vi "nanocal -- nuclear schottky fit V2.vi"() -> ()   [LabVIEW 2020]
uses:
  filename-pattern.ctl
  show-win- control.ctl
  cursor winow.ctl
  3-lorentzian-heat-response action.ctl
  nanocal-goodness-weighting-strategy.ctl
  <vilib>/gmath/NumericalOptimization/stopping criteria.ctl
  cursor window action.ctl
  cursor action.ctl
  2Dwindow.ctl
  publisher action.ctl
  <vilib>/gmath/NumericalOptimization/objective function data.ctl
  filename-action.ctl
  <vilib>/Utility/miscctls.llb/LVMapReplaceAction.ctl
  file -- read-write control.ctl
  array -- freq-voltage transformations action.ctl
  KM_file -- read-write control.ctl
  replace cursor action stack.vi
  Q -- range multiplier -- real -- V2.vi
  Q - not nan and gtr than zero - Real.vi
  Q - not nan -- real.vi
  Q -- check range -- i -- real.vi
  array - smart min max.vi
  3-lorentzian-heat-response -- V3.vi/142dd4c5-f9ed-c64b-bc14-a88e3e2c450a.vi
  3-lorentzian-heat-response -- analytic derivatives V3.vi
  array -- integrate scalar product.vi
  array -- freq-voltage transformations.vi/05c44075-957c-bc42-b6fa-2799d0bc0485.vi
  tale of three indices.vi
  filter -- window span logic.vi
  linear interp iiii- complex - z-omega - divide.vi
  linear interpolation iiii- complex.vi
  containing bix.vi
  3-lorentzian-heat-response.vi/142dd4c5-f9ed-c64b-bc14-a88e3e2c450a.vi
  <vilib>/Array/Sort 2D Array - Pop Stack.vi
  <vilib>/Array/Sort 2D Array - Push Stack.vi
  array -- freq-voltage transformations.vi/05c44075-957c-bc42-b6fa-2799d0bc0485.vi/5dd0d2be-718e-c148-b8fa-e083cdba2843.vi
  array -- freq-voltage transformations.vi/05c44075-957c-bc42-b6fa-2799d0bc0485.vi/095795a0-771d-c341-9fed-d90d2e44c51c.vi
  command stack.vi
  tale of three indices -- check state.vi
  Q -- check range -- i -- integer.vi
  linear interp iiii- complex - z-omega.vi
  line -- complex.vi
  Q - not nan -- integer.vi
  <vilib>/Analysis/baseanly.llb/A x B.vi
  <vilib>/Analysis/baseanly.llb/Complex A x B.vi
  array -- 3-finitediff.vi
  <vilib>/Analysis/polynomials.llb/Multiply Polynomials.vi
  <vilib>/Analysis/polynomials.llb/Multiply Polynomials (DBL).vi
  <vilib>/Analysis/polynomials.llb/Polynomial Roots.vi
  <vilib>/Analysis/polynomials.llb/Polynomial Roots (DBL).vi
  <vilib>/gmath/NumericalOptimization/Quasi Newton.vi
  <vilib>/Analysis/Matrix/Numeric/Conversions/Array To Matrix.vi
  <vilib>/Analysis/Matrix/Numeric/Conversions/Array To Matrix - RA2.vi
  <vilib>/Analysis/baseanly.llb/Inverse Matrix.vi
  <vilib>/Analysis/baseanly.llb/Real Inverse Matrix.vi
  <vilib>/Comparison/Less/Less Functor/Less Functor.lvclass
  <vilib>/gmath/NI_Gmath.lvlib
panel:
  in  "strings stuff tab":T1(tab)
  in  "string IN":string="  31 ->   <| \"ζ\"-> 0.003888489419  , \"τ1\"-> 0.087601168900  , \"τS\"-> 0.007032312731  , \"τN\"-> 0.055156103563  , \"τC\"-> 0.004551857108  , \"κ0\"-> 0.000000004997  , \"T\"-> 1.400000000000  , \"mm1\"-> 0.000000000000  , \"mm2\"-> 0.000000000000  , \"mm3\"-> 0.000000000000  , \"θ\"-> 0.000000000000  , \"B\"-> 35.000000000000  |>   , \r46 ->   <| \"ζ\"-> 0.005025241341  , \"τ1\"-> 0.102687516481  , \"τS\"-> 0.007383588614  , \"τN\"-> 0.103960168475  , \"τC\"-> 0.003866879432  , \"κ0\"-> 0.000000003907  , \"T\"-> 1.200000000000  , \"mm1\"-> 0.000000000000  , \"mm2\"-> 0.000000000000  , \"mm3\"-> 0.000000000000  , \"θ\"-> 0.000000000000  , \"B\"-> 35.000000000000  |>   , \r61 ->   <| \"ζ\"-> 0.005035416950  , \"τ1\"-> 0.122174929094  , \"τS\"-> 0.006222514600  , \"τN\"-> 0.205982547664  , \"τC\"-> 0.003366330966  , \"κ0\"-> 0.000000002719  , \"T\"-> 1.000000000000  , \"mm1\"-> 0.000000000000  , \"mm2\"-> 0.000000000000  , \"mm3\"-> 0.000000000000  , \"θ\"-> 0.000000000000  , \"B\"-> 35.000000000000  |>   , \r63 ->   <| \"ζ\"-> 0.005139197614  , \"τ1\"-> 0.198724796215  , \"τS\"-> 0.004800637014  , \"τN\"-> 0.465205171402  , \"τC\"-> 0.002863585191  , \"κ0\"-> 0.000000002155  , \"T\"-> 0.800000000000  , \"mm1\"-> 0.000000000000  , \"mm2\"-> 0.000000000000  , \"mm3\"-> 0.000000000000  , \"θ\"-> 0.000000000000  , \"B\"-> 35.000000000000  |>   , \r64 ->   <| \"ζ\"-> 0.004568953302  , \"τ1\"-> 0.093117776532  , \"τS\"-> 0.007355702079  , \"τN\"-> 0.062831572704  , \"τC\"-> 0.004650863735  , \"κ0\"-> 0.000000004736  , \"T\"-> 1.380000000000  , \"mm1\"-> 0.000000000000  , \"mm2\"-> 0.000000000000  , \"mm3\"-> 0.000000000000  , \"θ\"-> 0.000000000000  , \"B\"-> 35.000000000000  |>   , \r65 ->   <| \"ζ\"-> 0.002815263504  , \"τ1\"-> 0.065471361604  , \"τS\"-> 0.010801366154  , \"τN\"-> 0.021664996889  , \"τC\"-> 0.005770858189  , \"κ0\"-> 0.000000007227  , \"T\"-> 1.830000000000  , \"mm1\"-> 0.000000000000  , \"mm2\"-> 0.000000000000  , \"mm3\"-> 0.000000000000  , \"θ\"-> 0.000000000000  , \"B\"-> 35.000000000000  |>   , \r66 ->   <| \"ζ\"-> 0.002469190413  , \"τ1\"-> 0.040351968507  , \"τS\"-> 0.017885440476  , \"τN\"-> 0.005126718377  , \"τC\"-> 0.008463551777  , \"κ0\"-> 0.000000012143  , \"T\"-> 2.550000000000  , \"mm1\"-> 0.000000000000  , \"mm2\"-> 0.000000000000  , \"mm3\"-> 0.000000000000  , \"θ\"-> 0.000000000000  , \"B\"-> 35.000000000000  |>   , \r67 ->   <| \"ζ\"-> 0.003914938314  , \"τ1\"-> 0.009762017849  , \"τS\"-> 0.134374661960  , \"τN\"-> 0.000042356432  , \"τC\"-> 0.013647490504  , \"κ0\"-> 0.000000102341  , \"T\"-> 8.200000000000  , \"mm1\"-> 0.000048346937  , \"mm2\"-> 0.148545385808  , \"mm3\"-> 0.009759028335  , \"θ\"-> 0.000000000000  , \"B\"-> 35.000000000000  |>   , \r68 ->   <| \"ζ\"-> 0.006056953168  , \"τ1\"-> 0.011106014682  , \"τS\"-> 0.134857077980  , \"τN\"-> 0.000042354236  , \"τC\"-> 0.012982106024  , \"κ0\"-> 0.000000101776  , \"T\"-> 8.200000000000  , \"mm1\"-> 0.000000000000  , \"mm2\"-> 0.000000000000  , \"mm3\"-> 0.000000000000  , \"θ\"-> 0.000000000000  , \"B\"-> 25.000000000000  |>   , \r69 ->   <| \"ζ\"-> 0.003123114807  , \"τ1\"-> 0.020424162913  , \"τS\"-> 0.043527827747  , \"τN\"-> 0.000562268427  , \"τC\"-> 0.009966268738  , \"κ0\"-> 0.000000026661  , \"T\"-> 4.000000000000  , \"mm1\"-> 0.000000000000  , \"mm2\"-> 0.000000000000  , \"mm3\"-> 0.000000000000  , \"θ\"-> 0.000000000000  , \"B\"-> 35.000000000000  |>   , \r72 ->   <| \"ζ\"-> 0.002669122108  , \"τ1\"-> 0.038361259577  , \"τS\"-> 0.021199111100  , \"τN\"-> 0.003990494453  , \"τC\"-> 0.008668874028  , \"κ0\"-> 0.000000013704  , \"T\"-> 2.740000000000  , \"mm1\"-> 0.000000000000  , \"mm2\"-> 0.000000000000  , \"mm3\"-> 0.000000000000  , \"θ\"-> 0.000000000000  , \"B\"-> 35.000000000000  |>   , \r73 ->   <| \"ζ\"-> 0.002412108852  , \"τ1\"-> 0.040932774133  , \"τS\"-> 0.019260967968  , \"τN\"-> 0.005170470981  , \"τC\"-> 0.008253479704  , \"κ0\"-> 0.000000012614  , \"T\"-> 2.620000000000  , \"mm1\"-> 0.000000000000  , \"mm2\"-> 0.000000000000  , \"mm3\"-> 0.000000000000  , \"θ\"-> 0.000000000000  , \"B\"-> 35.000000000000  |>   , \r74 ->   <| \"ζ\"-> 0.002862853880  , \"τ1\"-> 0.054461176556  , \"τS\"-> 0.013607182187  , \"τN\"-> 0.011343205053  , \"τC\"-> 0.007225916211  , \"κ0\"-> 0.000000009324  , \"T\"-> 2.130000000000  , \"mm1\"-> 0.000000000000  , \"mm2\"-> 0.000000000000  , \"mm3\"-> 0.000000000000  , \"θ\"-> 0.000000000000  , \"B\"-> 35.000000000000  |>   , \r75 ->   <| \"ζ\"-> 0.003310560377  , \"τ1\"-> 0.073698198291  , \"τS\"-> 0.008858283837  , \"τN\"-> 0.033317244772  , \"τC\"-> 0.005489655620  , \"κ0\"-> 0.000000006041  , \"T\"-> 1.600000000000  , \"mm1\"-> 0.000000000000  , \"mm2\"-> 0.000000000000  , \"mm3\"-> 0.000000000000  , \"θ\"-> 0.000000000000  , \"B\"-> 35.000000000000  |>   , \r76 ->   <| \"ζ\"-> 0.004777415229  , \"τ1\"-> 0.096465030619  , \"τS\"-> 0.006885176015  , \"τN\"-> 0.081406405423  , \"τC\"-> 0.004205655089  , \"κ0\"-> 0.000000004144  , \"T\"-> 1.200000000000  , \"mm1\"-> 0.000000000000  , \"mm2\"-> 0.000000000000  , \"mm3\"-> 0.000000000000  , \"θ\"-> 0.000000000000  , \"B\"-> 35.000000000000  |>   , \r"
  in  "math -->   τ's !":bool
  in  "τ's --> math!":bool
  out "string OUT":string="  31 ->   <| \"ζ\"-> 0.003888489419  , \"τ1\"-> 0.087601168900  , \"τS\"-> 0.007032312731  , \"τN\"-> 0.055156103563  , \"τC\"-> 0.004551857108  , \"κ0\"-> 0.000000004997  , \"T\"-> 1.400000000000  , \"mm1\"-> 0.000000000000  , \"mm2\"-> 0.000000000000  , \"mm3\"-> 0.000000000000  , \"θ\"-> 0.000000000000  , \"B\"-> 35.000000000000  |>   , \r46 ->   <| \"ζ\"-> 0.005025241341  , \"τ1\"-> 0.102687516481  , \"τS\"-> 0.007383588614  , \"τN\"-> 0.103960168475  , \"τC\"-> 0.003866879432  , \"κ0\"-> 0.000000003907  , \"T\"-> 1.200000000000  , \"mm1\"-> 0.000000000000  , \"mm2\"-> 0.000000000000  , \"mm3\"-> 0.000000000000  , \"θ\"-> 0.000000000000  , \"B\"-> 35.000000000000  |>   , \r61 ->   <| \"ζ\"-> 0.005035416950  , \"τ1\"-> 0.122174929094  , \"τS\"-> 0.006222514600  , \"τN\"-> 0.205982547664  , \"τC\"-> 0.003366330966  , \"κ0\"-> 0.000000002719  , \"T\"-> 1.000000000000  , \"mm1\"-> 0.000000000000  , \"mm2\"-> 0.000000000000  , \"mm3\"-> 0.000000000000  , \"θ\"-> 0.000000000000  , \"B\"-> 35.000000000000  |>   , \r63 ->   <| \"ζ\"-> 0.005139197614  , \"τ1\"-> 0.198724796215  , \"τS\"-> 0.004800637014  , \"τN\"-> 0.465205171402  , \"τC\"-> 0.002863585191  , \"κ0\"-> 0.000000002155  , \"T\"-> 0.800000000000  , \"mm1\"-> 0.000000000000  , \"mm2\"-> 0.000000000000  , \"mm3\"-> 0.000000000000  , \"θ\"-> 0.000000000000  , \"B\"-> 35.000000000000  |>   , \r64 ->   <| \"ζ\"-> 0.004568953302  , \"τ1\"-> 0.093117776532  , \"τS\"-> 0.007355702079  , \"τN\"-> 0.062831572704  , \"τC\"-> 0.004650863735  , \"κ0\"-> 0.000000004736  , \"T\"-> 1.380000000000  , \"mm1\"-> 0.000000000000  , \"mm2\"-> 0.000000000000  , \"mm3\"-> 0.000000000000  , \"θ\"-> 0.000000000000  , \"B\"-> 35.000000000000  |>   , \r65 ->   <| \"ζ\"-> 0.002815263504  , \"τ1\"-> 0.065471361604  , \"τS\"-> 0.010801366154  , \"τN\"-> 0.021664996889  , \"τC\"-> 0.005770858189  , \"κ0\"-> 0.000000007227  , \"T\"-> 1.830000000000  , \"mm1\"-> 0.000000000000  , \"mm2\"-> 0.000000000000  , \"mm3\"-> 0.000000000000  , \"θ\"-> 0.000000000000  , \"B\"-> 35.000000000000  |>   , \r66 ->   <| \"ζ\"-> 0.002469190413  , \"τ1\"-> 0.040351968507  , \"τS\"-> 0.017885440476  , \"τN\"-> 0.005126718377  , \"τC\"-> 0.008463551777  , \"κ0\"-> 0.000000012143  , \"T\"-> 2.550000000000  , \"mm1\"-> 0.000000000000  , \"mm2\"-> 0.000000000000  , \"mm3\"-> 0.000000000000  , \"θ\"-> 0.000000000000  , \"B\"-> 35.000000000000  |>   , \r67 ->   <| \"ζ\"-> 0.003914938314  , \"τ1\"-> 0.009762017849  , \"τS\"-> 0.134374661960  , \"τN\"-> 0.000042356432  , \"τC\"-> 0.013647490504  , \"κ0\"-> 0.000000102341  , \"T\"-> 8.200000000000  , \"mm1\"-> 0.000048346937  , \"mm2\"-> 0.148545385808  , \"mm3\"-> 0.009759028335  , \"θ\"-> 0.000000000000  , \"B\"-> 35.000000000000  |>   , \r68 ->   <| \"ζ\"-> 0.006056953168  , \"τ1\"-> 0.011106014682  , \"τS\"-> 0.134857077980  , \"τN\"-> 0.000042354236  , \"τC\"-> 0.012982106024  , \"κ0\"-> 0.000000101776  , \"T\"-> 8.200000000000  , \"mm1\"-> 0.000000000000  , \"mm2\"-> 0.000000000000  , \"mm3\"-> 0.000000000000  , \"θ\"-> 0.000000000000  , \"B\"-> 25.000000000000  |>   , \r69 ->   <| \"ζ\"-> 0.003123114807  , \"τ1\"-> 0.020424162913  , \"τS\"-> 0.043527827747  , \"τN\"-> 0.000562268427  , \"τC\"-> 0.009966268738  , \"κ0\"-> 0.000000026661  , \"T\"-> 4.000000000000  , \"mm1\"-> 0.000000000000  , \"mm2\"-> 0.000000000000  , \"mm3\"-> 0.000000000000  , \"θ\"-> 0.000000000000  , \"B\"-> 35.000000000000  |>   , \r72 ->   <| \"ζ\"-> 0.002669122108  , \"τ1\"-> 0.038361259577  , \"τS\"-> 0.021199111100  , \"τN\"-> 0.003990494453  , \"τC\"-> 0.008668874028  , \"κ0\"-> 0.000000013704  , \"T\"-> 2.740000000000  , \"mm1\"-> 0.000000000000  , \"mm2\"-> 0.000000000000  , \"mm3\"-> 0.000000000000  , \"θ\"-> 0.000000000000  , \"B\"-> 35.000000000000  |>   , \r73 ->   <| \"ζ\"-> 0.002412108852  , \"τ1\"-> 0.040932774133  , \"τS\"-> 0.019260967968  , \"τN\"-> 0.005170470981  , \"τC\"-> 0.008253479704  , \"κ0\"-> 0.000000012614  , \"T\"-> 2.620000000000  , \"mm1\"-> 0.000000000000  , \"mm2\"-> 0.000000000000  , \"mm3\"-> 0.000000000000  , \"θ\"-> 0.000000000000  , \"B\"-> 35.000000000000  |>   , \r74 ->   <| \"ζ\"-> 0.002862853880  , \"τ1\"-> 0.054461176556  , \"τS\"-> 0.013607182187  , \"τN\"-> 0.011343205053  , \"τC\"-> 0.007225916211  , \"κ0\"-> 0.000000009324  , \"T\"-> 2.130000000000  , \"mm1\"-> 0.000000000000  , \"mm2\"-> 0.000000000000  , \"mm3\"-> 0.000000000000  , \"θ\"-> 0.000000000000  , \"B\"-> 35.000000000000  |>   , \r75 ->   <| \"ζ\"-> 0.003310560377  , \"τ1\"-> 0.073698198291  , \"τS\"-> 0.008858283837  , \"τN\"-> 0.033317244772  , \"τC\"-> 0.005489655620  , \"κ0\"-> 0.000000006041  , \"T\"-> 1.600000000000  , \"mm1\"-> 0.000000000000  , \"mm2\"-> 0.000000000000  , \"mm3\"-> 0.000000000000  , \"θ\"-> 0.000000000000  , \"B\"-> 35.000000000000  |>   , \r76 ->   <| \"ζ\"-> 0.004777415229  , \"τ1\"-> 0.096465030619  , \"τS\"-> 0.006885176015  , \"τN\"-> 0.081406405423  , \"τC\"-> 0.004205655089  , \"κ0\"-> 0.000000004144  , \"T\"-> 1.200000000000  , \"mm1\"-> 0.000000000000  , \"mm2\"-> 0.000000000000  , \"mm3\"-> 0.000000000000  , \"θ\"-> 0.000000000000  , \"B\"-> 35.000000000000  |>   , \r"
  in  "math --> string!":bool
  in  "string --> math!":bool
  in  "file pattern":string="Indium_June2021_*_ark.dat"
  in  "folder":path=path "/opt/new/Dropbox/desktop_data/Indium-nanocal-cell12-June2021/labview-ready-files"
  in  "filenames":u16(ring)=13 caption="files" items=["CeCoIn5_2nd_071_12T_0.120K_90deg_fdep_labview_.dat", "CeCoIn5_2nd_048_12T_0.148K_0deg_freqDep_labview_.dat", "CeCoIn5_2nd_072_12T_0.148K_90deg_fdep_labview_.dat", "CeCoIn5_2nd_049_12T_0.179K_0deg_freqDep_labview_.dat", "CeCoIn5_2nd_070_12T_0.179K_90deg_fdep_labview_.dat", "CeCoIn5_2nd_050_12T_0.197K_0deg_freqDep_labview_.dat", "CeCoIn5_2nd_073_12T_0.197K_90deg_fdep_labview_.dat", "CeCoIn5_2nd_074_12T_0.249K_90deg_fdep_labview_.dat", "CeCoIn5_2nd_051_12T_0.25K_0deg_freqDep_labview_.dat", "CeCoIn5_2nd_052_12T_0.3K_0deg_freqDep_labview_.dat", "CeCoIn5_2nd_075_12T_0.300K_90deg_fdep_labview_.dat", "CeCoIn5_2nd_053_12T_0.360K_0deg_freqDep_labview_.dat", "CeCoIn5_2nd_076_12T_0.360K_90deg_fdep_labview_.dat", "CeCoIn5_2nd_054_12T_0.430K_0deg_freqDep_labview_.dat", "CeCoIn5_2nd_077_12T_0.430K_90deg_fdep_labview_.dat", "CeCoIn5_2nd_055_12T_0.512K_0deg_freqDep_labview_.dat", "CeCoIn5_2nd_078_12T_0.512K_90deg_fdep_labview_.dat", "CeCoIn5_2nd_056_12T_0.61K_0deg_freqDep_labview_.dat", "CeCoIn5_2nd_079_12T_0.610K_90deg_fdep_labview_.dat", "CeCoIn5_2nd_057_12T_0.81K_0deg_freqDep_labview_.dat", "CeCoIn5_2nd_080_12T_0.810K_90deg_fdep_labview_.dat", "CeCoIn5_2nd_081_12T_1.1K_90deg_fdep_labview_.dat", "CeCoIn5_2nd_058_12T_1.12K_0deg_freqDep_labview_.dat", "CeCoIn5_2nd_059_12T_1.8K_0deg_freqDep_labview_.dat", "CeCoIn5_2nd_082_12T_1.8K_90deg_fdep_labview_.dat", "CeCoIn5_2nd_060_12T_3.0K_0deg_freqDep_labview_.dat", "CeCoIn5_2nd_083_12T_3.0K_90deg_fdep_labview_.dat", "CeCoIn5_2nd_061_12T_5.5K_0deg_freqDep_labview_.dat", "CeCoIn5_2nd_084_12T_5.7K_90deg_fdep_labview_.dat"]
  out "notes":string="  48 ->   <| \"ζ\"-> 0.225182112153  , \"τ1\"-> 0.030427185371  , \"τS\"-> 0.215756406989  , \"τN\"-> 0.297516075068  , \"τC\"-> 0.001159880124  , \"κ0\"-> 0.000000000757  , \"T\"-> 0.148000000000  , \"mm1\"-> 0.000000000000  , \"mm2\"-> 0.000000000000  , \"mm3\"-> 0.000000000000  , \"θ\"-> 0.000000000000  |>   , \r49 ->   <| \"ζ\"-> 0.172076901868  , \"τ1\"-> 0.029034369734  , \"τS\"-> 0.155813864567  , \"τN\"-> 0.144653734876  , \"τC\"-> 0.001114471886  , \"κ0\"-> 0.000000001041  , \"T\"-> 0.179000000000  , \"mm1\"-> 0.000000000000  , \"mm2\"-> 0.000000000000  , \"mm3\"-> 0.000000000000  , \"θ\"-> 0.000000000000  |>   , \r50 ->   <| \"ζ\"-> 0.148077728243  , \"τ1\"-> 0.028544607399  , \"τS\"-> 0.124620640187  , \"τN\"-> 0.093757074751  , \"τC\"-> 0.001082877171  , \"κ0\"-> 0.000000001180  , \"T\"-> 0.197000000000  , \"mm1\"-> 0.000000000000  , \"mm2\"-> 0.000000000000  , \"mm3\"-> 0.000000000000  , \"θ\"-> 0.000000000000  |>   , \r51 ->   <| \"ζ\"-> 0.081193222097  , \"τ1\"-> 0.024715806431  , \"τS\"-> 0.089455978355  , \"τN\"-> 0.032053841538  , \"τC\"-> 0.001544599185  , \"κ0\"-> 0.000000001536  , \"T\"-> 0.250000000000  , \"mm1\"-> 0.000000000000  , \"mm2\"-> 0.000000000000  , \"mm3\"-> 0.000000000000  , \"θ\"-> 0.000000000000  |>   , \r52 ->   <| \"ζ\"-> 0.048082496373  , \"τ1\"-> 0.022642786515  , \"τS\"-> 0.068869549235  , \"τN\"-> 0.016486235683  , \"τC\"-> 0.002476229885  , \"κ0\"-> 0.000000001973  , \"T\"-> 0.300000000000  , \"mm1\"-> 0.000000000000  , \"mm2\"-> 0.000000000000  , \"mm3\"-> 0.000000000000  , \"θ\"-> 0.000000000000  |>   , \r53 ->   <| \"ζ\"-> 0.038407326202  , \"τ1\"-> 0.020371560008  , \"τS\"-> 0.055508745241  , \"τN\"-> 0.008451508810  , \"τC\"-> 0.002530832197  , \"κ0\"-> 0.000000002423  , \"T\"-> 0.360000000000  , \"mm1\"-> 0.000000000000  , \"mm2\"-> 0.000000000000  , \"mm3\"-> 0.000000000000  , \"θ\"-> 0.000000000000  |>   , \r54 ->   <| \"ζ\"-> 0.025817013343  , \"τ1\"-> 0.018385471103  , \"τS\"-> 0.045747558757  , \"τN\"-> 0.005165003032  , \"τC\"-> 0.002680275541  , \"κ0\"-> 0.000000002982  , \"T\"-> 0.430000000000  , \"mm1\"-> 0.000000000000  , \"mm2\"-> 0.000000000000  , \"mm3\"-> 0.000000000000  , \"θ\"-> 0.000000000000  |>   , \r55 ->   <| \"ζ\"-> 0.019908376980  , \"τ1\"-> 0.016902177597  , \"τS\"-> 0.037431350421  , \"τN\"-> 0.003115611581  , \"τC\"-> 0.002813000351  , \"κ0\"-> 0.000000003723  , \"T\"-> 0.512000000000  , \"mm1\"-> 0.000000000000  , \"mm2\"-> 0.000000000000  , \"mm3\"-> 0.000000000000  , \"θ\"-> 0.000000000000  |>   , \r56 ->   <| \"ζ\"-> 0.018376000000  , \"τ1\"-> 0.014989979497  , \"τS\"-> 0.031364970092  , \"τN\"-> 0.001876083588  , \"τC\"-> 0.004034409107  , \"κ0\"-> 0.000000004410  , \"T\"-> 0.610000000000  , \"mm1\"-> 0.000000000000  , \"mm2\"-> 0.000000000000  , \"mm3\"-> 0.000000000000  , \"θ\"-> 0.000000000000  |>   , \r57 ->   <| \"ζ\"-> 0.015651665128  , \"τ1\"-> 0.013298894889  , \"τS\"-> 0.022882494925  , \"τN\"-> 0.000826522678  , \"τC\"-> 0.005306542804  , \"κ0\"-> 0.000000006075  , \"T\"-> 0.810000000000  , \"mm1\"-> 0.000000000000  , \"mm2\"-> 0.000000000000  , \"mm3\"-> 0.000000000000  , \"θ\"-> 0.000000000000  |>   , \r58 ->   <| \"ζ\"-> 0.011916480594  , \"τ1\"-> 0.012551282481  , \"τS\"-> 0.018233218660  , \"τN\"-> 0.000345702746  , \"τC\"-> 0.004699451527  , \"κ0\"-> 0.000000008451  , \"T\"-> 1.120000000000  , \"mm1\"-> 0.000000000000  , \"mm2\"-> 0.000000000000  , \"mm3\"-> 0.000000000000  , \"θ\"-> 0.000000000000  |>   , \r59 ->   <| \"ζ\"-> 0.012831327568  , \"τ1\"-> 0.013315909415  , \"τS\"-> 0.012590836847  , \"τN\"-> 0.000065003013  , \"τC\"-> 0.005276356243  , \"κ0\"-> 0.000000013610  , \"T\"-> 1.800000000000  , \"mm1\"-> 0.000000000000  , \"mm2\"-> 0.000000000000  , \"mm3\"-> 0.000000000000  , \"θ\"-> 0.000000000000  |>   , \r60 ->   <| \"ζ\"-> 0.019774146838  , \"τ1\"-> 0.013257273421  , \"τS\"-> 0.007064131508  , \"τN\"-> 0.000028000819  , \"τC\"-> 0.006942241845  , \"κ0\"-> 0.000000023477  , \"T\"-> 3.000000000000  , \"mm1\"-> 0.000000000000  , \"mm2\"-> 0.000000000000  , \"mm3\"-> 0.000000000000  , \"θ\"-> 0.000000000000  |>   , \r61 ->   <| \"ζ\"-> 0.029251354442  , \"τ1\"-> 0.014634751206  , \"τS\"-> 0.003873958746  , \"τN\"-> 0.000007000487  , \"τC\"-> 0.006827504775  , \"κ0\"-> 0.000000056438  , \"T\"-> 5.500000000000  , \"mm1\"-> 0.000000000000  , \"mm2\"-> 0.000000000000  , \"mm3\"-> 0.000000000000  , \"θ\"-> 0.000000000000  |>   , \r70 ->   <| \"ζ\"-> 0.160286026344  , \"τ1\"-> 0.073452047785  , \"τS\"-> 0.044872374187  , \"τN\"-> 0.162076895387  , \"τC\"-> 0.001481759328  , \"κ0\"-> 0.000000001039  , \"T\"-> 0.179000000000  , \"mm1\"-> 0.000000000000  , \"mm2\"-> 0.000000000000  , \"mm3\"-> 0.000000000000  , \"θ\"-> 90.000000000000  |>   , \r71 ->   <| \"ζ\"-> 0.317192968490  , \"τ1\"-> 0.095324848000  , \"τS\"-> 0.087097785701  , \"τN\"-> 0.936221653169  , \"τC\"-> 0.001480807262  , \"κ0\"-> 0.000000000534  , \"T\"-> 0.120000000000  , \"mm1\"-> 0.000000000000  , \"mm2\"-> 0.000000000000  , \"mm3\"-> 0.000000000000  , \"θ\"-> 90.000000000000  |>   , \r72 ->   <| \"ζ\"-> 0.222764630124  , \"τ1\"-> 0.096058032825  , \"τS\"-> 0.066495942806  , \"τN\"-> 0.366151877245  , \"τC\"-> 0.001319275999  , \"κ0\"-> 0.000000000769  , \"T\"-> 0.148000000000  , \"mm1\"-> 0.000000000000  , \"mm2\"-> 0.000000000000  , \"mm3\"-> 0.000000000000  , \"θ\"-> 90.000000000000  |>   , \r73 ->   <| \"ζ\"-> 0.136082903087  , \"τ1\"-> 0.070214285183  , \"τS\"-> 0.041562366618  , \"τN\"-> 0.122478563978  , \"τC\"-> 0.001561716081  , \"κ0\"-> 0.000000001214  , \"T\"-> 0.197000000000  , \"mm1\"-> 0.000000000000  , \"mm2\"-> 0.000000000000  , \"mm3\"-> 0.000000000000  , \"θ\"-> 90.000000000000  |>   , \r74 ->   <| \"ζ\"-> 0.079924133870  , \"τ1\"-> 0.053892600038  , \"τS\"-> 0.033721986821  , \"τN\"-> 0.048194390820  , \"τC\"-> 0.001786420268  , \"κ0\"-> 0.000000001543  , \"T\"-> 0.249000000000  , \"mm1\"-> 0.000000000000  , \"mm2\"-> 0.000000000000  , \"mm3\"-> 0.000000000000  , \"θ\"-> 90.000000000000  |>   , \r75 ->   <| \"ζ\"-> 0.055680730504  , \"τ1\"-> 0.044845519236  , \"τS\"-> 0.029550773155  , \"τN\"-> 0.023428217313  , \"τC\"-> 0.002197475136  , \"κ0\"-> 0.000000001960  , \"T\"-> 0.300000000000  , \"mm1\"-> 0.000000000000  , \"mm2\"-> 0.000000000000  , \"mm3\"-> 0.000000000000  , \"θ\"-> 90.000000000000  |>   , \r76 ->   <| \"ζ\"-> 0.040648812263  , \"τ1\"-> 0.038083560479  , \"τS\"-> 0.026574795079  , \"τN\"-> 0.013361826633  , \"τC\"-> 0.002899405432  , \"κ0\"-> 0.000000002383  , \"T\"-> 0.360000000000  , \"mm1\"-> 0.000000000000  , \"mm2\"-> 0.000000000000  , \"mm3\"-> 0.000000000000  , \"θ\"-> 90.000000000000  |>   , \r77 ->   <| \"ζ\"-> 0.031873906103  , \"τ1\"-> 0.030223838950  , \"τS\"-> 0.024286132427  , \"τN\"-> 0.006926780152  , \"τC\"-> 0.002978043437  , \"κ0\"-> 0.000000002967  , \"T\"-> 0.430000000000  , \"mm1\"-> 0.000000000000  , \"mm2\"-> 0.000000000000  , \"mm3\"-> 0.000000000000  , \"θ\"-> 90.000000000000  |>   , \r78 ->   <| \"ζ\"-> 0.025948172116  , \"τ1\"-> 0.025051552712  , \"τS\"-> 0.022571188655  , \"τN\"-> 0.003812228812  , \"τC\"-> 0.003259730052  , \"κ0\"-> 0.000000003686  , \"T\"-> 0.512000000000  , \"mm1\"-> 0.000000000000  , \"mm2\"-> 0.000000000000  , \"mm3\"-> 0.000000000000  , \"θ\"-> 90.000000000000  |>   , \r79 ->   <| \"ζ\"-> 0.020946044060  , \"τ1\"-> 0.024756174566  , \"τS\"-> 0.021099556284  , \"τN\"-> 0.002276701384  , \"τC\"-> 0.004159440288  , \"κ0\"-> 0.000000004389  , \"T\"-> 0.610000000000  , \"mm1\"-> 0.000000000000  , \"mm2\"-> 0.000000000000  , \"mm3\"-> 0.000000000000  , \"θ\"-> 90.000000000000  |>   , \r80 ->   <| \"ζ\"-> 0.014774082145  , \"τ1\"-> 0.015773102766  , \"τS\"-> 0.018723894921  , \"τN\"-> 0.000790199963  , \"τC\"-> 0.005097561693  , \"κ0\"-> 0.000000006095  , \"T\"-> 0.810000000000  , \"mm1\"-> 0.000000000000  , \"mm2\"-> 0.000000000000  , \"mm3\"-> 0.000000000000  , \"θ\"-> 90.000000000000  |>   , \r81 ->   <| \"ζ\"-> 0.013971175207  , \"τ1\"-> 0.015831825440  , \"τS\"-> 0.017293056061  , \"τN\"-> 0.000406001835  , \"τC\"-> 0.005061653181  , \"κ0\"-> 0.000000008423  , \"T\"-> 1.100000000000  , \"mm1\"-> 0.000000000000  , \"mm2\"-> 0.000000000000  , \"mm3\"-> 0.000000000000  , \"θ\"-> 90.000000000000  |>   , \r82 ->   <| \"ζ\"-> 0.014703834330  , \"τ1\"-> 0.019025451961  , \"τS\"-> 0.011790469569  , \"τN\"-> 0.000107003492  , \"τC\"-> 0.007625608278  , \"κ0\"-> 0.000000014259  , \"T\"-> 1.800000000000  , \"mm1\"-> 0.000000000000  , \"mm2\"-> 0.000000000000  , \"mm3\"-> 0.000000000000  , \"θ\"-> 90.000000000000  |>   , \r83 ->   <| \"ζ\"-> 0.021950059397  , \"τ1\"-> 0.019029879523  , \"τS\"-> 0.006582834729  , \"τN\"-> 0.000028012011  , \"τC\"-> 0.009051896214  , \"κ0\"-> 0.000000024750  , \"T\"-> 3.000000000000  , \"mm1\"-> 0.000000000000  , \"mm2\"-> 0.000000000000  , \"mm3\"-> 0.000000000000  , \"θ\"-> 90.000000000000  |>   , \r84 ->   <| \"ζ\"-> 0.027897403691  , \"τ1\"-> 0.014639690770  , \"τS\"-> 0.004105291179  , \"τN\"-> 0.000006999171  , \"τC\"-> 0.007414449545  , \"κ0\"-> 0.000000059701  , \"T\"-> 5.700000000000  , \"mm1\"-> 0.000073450671  , \"mm2\"-> 0.014673310812  , \"mm3\"-> 0.011534391407  , \"θ\"-> 90.000000000000  |>   , \r"
  in  "mathematica thing":map{i32, map{T2, dbl}}(c390)={31={enum."dζ"=0.003888489419, enum."dT1"=0.0876011689, enum."dτS"=0.007032312731, enum."dτN"=0.055156103563, enum."dτC"=0.004551857108, enum."dκ0"=4.997e-09, enum."T(K)"=1.4, enum."θ (deg)"=0.0, enum."B (T)"=35.0}, 46={enum."dζ"=0.005025241341, enum."dT1"=0.102687516481, enum."dτS"=0.007383588614, enum."dτN"=0.103960168475, enum."dτC"=0.003866879432, enum."dκ0"=3.907e-09, enum."T(K)"=1.2, enum."θ (deg)"=0.0, enum."B (T)"=35.0}, 61={enum."dζ"=0.00503541695, enum."dT1"=0.122174929094, enum."dτS"=0.0062225146, enum."dτN"=0.205982547664, enum."dτC"=0.003366330966, enum."dκ0"=2.719e-09, enum."T(K)"=1.0, enum."θ (deg)"=0.0, enum."B (T)"=35.0}, 63={enum."dζ"=0.005139197614, enum."dT1"=0.198724796215, enum."dτS"=0.004800637014, enum."dτN"=0.465205171402, enum."dτC"=0.002863585191, enum."dκ0"=2.155e-09, enum."T(K)"=0.8, enum."θ (deg)"=0.0, enum."B (T)"=35.0}, 64={enum."dζ"=0.004568953302, enum."dT1"=0.093117776532, enum."dτS"=0.007355702079, enum."dτN"=0.062831572704, enum."dτC"=0.004650863735, enum."dκ0"=4.736e-09, enum."T(K)"=1.38, enum."θ (deg)"=0.0, enum."B (T)"=35.0}, 65={enum."dζ"=0.002815263504, enum."dT1"=0.065471361604, enum."dτS"=0.010801366154, enum."dτN"=0.021664996889, enum."dτC"=0.005770858189, enum."dκ0"=7.227e-09, enum."T(K)"=1.83, enum."θ (deg)"=0.0, enum."B (T)"=35.0}, 66={enum."dζ"=0.002469190413, enum."dT1"=0.040351968507, enum."dτS"=0.017885440476, enum."dτN"=0.005126718377, enum."dτC"=0.008463551777, enum."dκ0"=1.2143e-08, enum."T(K)"=2.55, enum."θ (deg)"=0.0, enum."B (T)"=35.0}, 67={enum."dζ"=0.00391493831404709, enum."dT1"=0.009762017848695768, enum."dτS"=0.13437466196040418, enum."dτN"=4.235643214853134e-05, enum."dτC"=0.013647490503661961, enum."dκ0"=1.0234079529926423e-07, enum."T(K)"=8.2, enum."m1"=4.8346936616345945e-05, enum."m2"=0.14854538580834648, enum."m3"=0.009759028335312583, enum."θ (deg)"=0.0, enum."B (T)"=35.0}, 68={enum."dζ"=0.006056953168, enum."dT1"=0.011106014682, enum."dτS"=0.13485707798, enum."dτN"=4.2354236e-05, enum."dτC"=0.012982106024, enum."dκ0"=1.01776e-07, enum."T(K)"=8.2, enum."θ (deg)"=0.0, enum."B (T)"=25.0}, 69={enum."dζ"=0.003123114807, enum."dT1"=0.020424162913, enum."dτS"=0.043527827747, enum."dτN"=0.000562268427, enum."dτC"=0.009966268738, enum."dκ0"=2.6661e-08, enum."T(K)"=4.0, enum."θ (deg)"=0.0, enum."B (T)"=35.0}, 72={enum."dζ"=0.002669122108, enum."dT1"=0.038361259577, enum."dτS"=0.0211991111, enum."dτN"=0.003990494453, enum."dτC"=0.008668874028, enum."dκ0"=1.3704e-08, enum."T(K)"=2.74, enum."θ (deg)"=0.0, enum."B (T)"=35.0}, 73={enum."dζ"=0.002412108852, enum."dT1"=0.040932774133, enum."dτS"=0.019260967968, enum."dτN"=0.005170470981, enum."dτC"=0.008253479704, enum."dκ0"=1.2614e-08, enum."T(K)"=2.62, enum."θ (deg)"=0.0, enum."B (T)"=35.0}, 74={enum."dζ"=0.00286285388, enum."dT1"=0.054461176556, enum."dτS"=0.013607182187, enum."dτN"=0.011343205053, enum."dτC"=0.007225916211, enum."dκ0"=9.324e-09, enum."T(K)"=2.13, enum."θ (deg)"=0.0, enum."B (T)"=35.0}, 75={enum."dζ"=0.003310560377, enum."dT1"=0.073698198291, enum."dτS"=0.008858283837, enum."dτN"=0.033317244772, enum."dτC"=0.00548965562, enum."dκ0"=6.041e-09, enum."T(K)"=1.6, enum."θ (deg)"=0.0, enum."B (T)"=35.0}, 76={enum."dζ"=0.004777415229, enum."dT1"=0.096465030619, enum."dτS"=0.006885176015, enum."dτN"=0.081406405423, enum."dτC"=0.004205655089, enum."dκ0"=4.144e-09, enum."T(K)"=1.2, enum."θ (deg)"=0.0, enum."B (T)"=35.0}}
  out "filenames":map{i32, string}(c390)={31="Indium_June2021_031_1.4K_35T_sh_ark.dat", 46="Indium_June2021_046_1.2K_35T_sh_ark.dat", 61="Indium_June2021_061_1.0K_35T_dc_sh_ark.dat", 63="Indium_June2021_063_0.8K_35T_dc_sh_ark.dat", 64="Indium_June2021_064_1.38K_35T_dc_sh_ark.dat", 65="Indium_June2021_065_1.83K_35T_dc_sh_ark.dat", 66="Indium_June2021_066_2.55K_35T_dc_sh_ark.dat", 67="Indium_June2021_067_8.2K_35T_dc_sh_ark.dat", 68="Indium_June2021_068_8.2K_25T_dc_sh_ark.dat", 69="Indium_June2021_069_4K_35T_dc_sh_ark.dat", 72="Indium_June2021_072_2.74K_35T_dc_sh_ark.dat", 73="Indium_June2021_073_2.62K_35T_dc_sh_ark.dat", 74="Indium_June2021_074_2.13K_35T_dc_sh_ark.dat", 75="Indium_June2021_075_1.6K_35T_dc_sh_ark.dat", 76="Indium_June2021_076_1.2K_35T_dc_sh_ark.dat"}
  out "temps&degs":map{i32, map{T2, dbl}}(c390)={31={enum."T(K)"=1.4, enum."θ (deg)"=0.0, enum."B (T)"=35.0}, 46={enum."T(K)"=1.2, enum."θ (deg)"=0.0, enum."B (T)"=35.0}, 61={enum."T(K)"=1.0, enum."θ (deg)"=0.0, enum."B (T)"=35.0}, 63={enum."T(K)"=0.8, enum."θ (deg)"=0.0, enum."B (T)"=35.0}, 64={enum."T(K)"=1.38, enum."θ (deg)"=0.0, enum."B (T)"=35.0}, 65={enum."T(K)"=1.83, enum."θ (deg)"=0.0, enum."B (T)"=35.0}, 66={enum."T(K)"=2.55, enum."θ (deg)"=0.0, enum."B (T)"=35.0}, 67={enum."T(K)"=8.2, enum."θ (deg)"=0.0, enum."B (T)"=35.0}, 68={enum."T(K)"=8.2, enum."θ (deg)"=0.0, enum."B (T)"=25.0}, 69={enum."T(K)"=4.0, enum."θ (deg)"=0.0, enum."B (T)"=35.0}, 72={enum."T(K)"=2.74, enum."θ (deg)"=0.0, enum."B (T)"=35.0}, 73={enum."T(K)"=2.62, enum."θ (deg)"=0.0, enum."B (T)"=35.0}, 74={enum."T(K)"=2.13, enum."θ (deg)"=0.0, enum."B (T)"=35.0}, 75={enum."T(K)"=1.6, enum."θ (deg)"=0.0, enum."B (T)"=35.0}, 76={enum."T(K)"=1.2, enum."θ (deg)"=0.0, enum."B (T)"=35.0}}
  out "cursor x selector":map{T2, dbl}(c390)={enum."T(K)"=8.2, enum."θ (deg)"=0.0, enum."B (T)"=35.0}
  out "Set of B's":set{dbl}(c389)={25.0, 35.0}
  out "Set of θ's":set{dbl}(c389)
  out "Set of T's":set{dbl}(c389)={0.8, 1.0, 1.2, 1.38, 1.4, 1.6, 1.83, 2.13, 2.55, 2.62, 2.74, 4.0, 8.2}
  out "B lookup":map{i32, dbl}(c390)={0=25.0, 1=35.0}
  out "filesnames lookup":map{i32, i32}(c390)={0=63, 1=61, 2=46, 3=76, 4=64, 5=31, 6=75, 7=65, 8=74, 9=66, 10=73, 11=72, 12=69, 13=67, 14=68}
  out "θ lookup":map{i32, dbl}(c390)={0=0.0}
  out "T lookup":map{i32, dbl}(c390)={0=0.8, 1=1.0, 2=1.2, 3=1.38, 4=1.4, 5=1.6, 6=1.83, 7=2.13, 8=2.55, 9=2.62, 10=2.74, 11=4.0, 12=8.2}
  out "backup mathematica string OUT backup":string="  48 ->   <| \"ζ\"-> 0.225182112153  , \"τ1\"-> 0.030427185371  , \"τS\"-> 0.215756406989  , \"τN\"-> 0.297516075068  , \"τC\"-> 0.001159880124  , \"κ0\"-> 0.000000000757  , \"T\"-> 0.148000000000  , \"mm1\"-> 0.000000000000  , \"mm2\"-> 0.000000000000  , \"mm3\"-> 0.000000000000  , \"θ\"-> 0.000000000000  |>   , \r49 ->   <| \"ζ\"-> 0.172076901868  , \"τ1\"-> 0.029034369734  , \"τS\"-> 0.155813864567  , \"τN\"-> 0.144653734876  , \"τC\"-> 0.001114471886  , \"κ0\"-> 0.000000001041  , \"T\"-> 0.179000000000  , \"mm1\"-> 0.000000000000  , \"mm2\"-> 0.000000000000  , \"mm3\"-> 0.000000000000  , \"θ\"-> 0.000000000000  |>   , \r50 ->   <| \"ζ\"-> 0.148077728243  , \"τ1\"-> 0.028544607399  , \"τS\"-> 0.124620640187  , \"τN\"-> 0.093757074751  , \"τC\"-> 0.001082877171  , \"κ0\"-> 0.000000001180  , \"T\"-> 0.197000000000  , \"mm1\"-> 0.000000000000  , \"mm2\"-> 0.000000000000  , \"mm3\"-> 0.000000000000  , \"θ\"-> 0.000000000000  |>   , \r51 ->   <| \"ζ\"-> 0.081193222097  , \"τ1\"-> 0.024715806431  , \"τS\"-> 0.089455978355  , \"τN\"-> 0.032053841538  , \"τC\"-> 0.001544599185  , \"κ0\"-> 0.000000001536  , \"T\"-> 0.250000000000  , \"mm1\"-> 0.000000000000  , \"mm2\"-> 0.000000000000  , \"mm3\"-> 0.000000000000  , \"θ\"-> 0.000000000000  |>   , \r52 ->   <| \"ζ\"-> 0.048082496373  , \"τ1\"-> 0.022642786515  , \"τS\"-> 0.068869549235  , \"τN\"-> 0.016486235683  , \"τC\"-> 0.002476229885  , \"κ0\"-> 0.000000001973  , \"T\"-> 0.300000000000  , \"mm1\"-> 0.000000000000  , \"mm2\"-> 0.000000000000  , \"mm3\"-> 0.000000000000  , \"θ\"-> 0.000000000000  |>   , \r53 ->   <| \"ζ\"-> 0.038407326202  , \"τ1\"-> 0.020371560008  , \"τS\"-> 0.055508745241  , \"τN\"-> 0.008451508810  , \"τC\"-> 0.002530832197  , \"κ0\"-> 0.000000002423  , \"T\"-> 0.360000000000  , \"mm1\"-> 0.000000000000  , \"mm2\"-> 0.000000000000  , \"mm3\"-> 0.000000000000  , \"θ\"-> 0.000000000000  |>   , \r54 ->   <| \"ζ\"-> 0.025817013343  , \"τ1\"-> 0.018385471103  , \"τS\"-> 0.045747558757  , \"τN\"-> 0.005165003032  , \"τC\"-> 0.002680275541  , \"κ0\"-> 0.000000002982  , \"T\"-> 0.430000000000  , \"mm1\"-> 0.000000000000  , \"mm2\"-> 0.000000000000  , \"mm3\"-> 0.000000000000  , \"θ\"-> 0.000000000000  |>   , \r55 ->   <| \"ζ\"-> 0.019908376980  , \"τ1\"-> 0.016902177597  , \"τS\"-> 0.037431350421  , \"τN\"-> 0.003115611581  , \"τC\"-> 0.002813000351  , \"κ0\"-> 0.000000003723  , \"T\"-> 0.512000000000  , \"mm1\"-> 0.000000000000  , \"mm2\"-> 0.000000000000  , \"mm3\"-> 0.000000000000  , \"θ\"-> 0.000000000000  |>   , \r56 ->   <| \"ζ\"-> 0.018376000000  , \"τ1\"-> 0.014989979497  , \"τS\"-> 0.031364970092  , \"τN\"-> 0.001876083588  , \"τC\"-> 0.004034409107  , \"κ0\"-> 0.000000004410  , \"T\"-> 0.610000000000  , \"mm1\"-> 0.000000000000  , \"mm2\"-> 0.000000000000  , \"mm3\"-> 0.000000000000  , \"θ\"-> 0.000000000000  |>   , \r57 ->   <| \"ζ\"-> 0.015651665128  , \"τ1\"-> 0.013298894889  , \"τS\"-> 0.022882494925  , \"τN\"-> 0.000826522678  , \"τC\"-> 0.005306542804  , \"κ0\"-> 0.000000006075  , \"T\"-> 0.810000000000  , \"mm1\"-> 0.000000000000  , \"mm2\"-> 0.000000000000  , \"mm3\"-> 0.000000000000  , \"θ\"-> 0.000000000000  |>   , \r58 ->   <| \"ζ\"-> 0.011916480594  , \"τ1\"-> 0.012551282481  , \"τS\"-> 0.018233218660  , \"τN\"-> 0.000345702746  , \"τC\"-> 0.004699451527  , \"κ0\"-> 0.000000008451  , \"T\"-> 1.120000000000  , \"mm1\"-> 0.000000000000  , \"mm2\"-> 0.000000000000  , \"mm3\"-> 0.000000000000  , \"θ\"-> 0.000000000000  |>   , \r59 ->   <| \"ζ\"-> 0.012831327568  , \"τ1\"-> 0.013315909415  , \"τS\"-> 0.012590836847  , \"τN\"-> 0.000065003013  , \"τC\"-> 0.005276356243  , \"κ0\"-> 0.000000013610  , \"T\"-> 1.800000000000  , \"mm1\"-> 0.000000000000  , \"mm2\"-> 0.000000000000  , \"mm3\"-> 0.000000000000  , \"θ\"-> 0.000000000000  |>   , \r60 ->   <| \"ζ\"-> 0.019774146838  , \"τ1\"-> 0.013257273421  , \"τS\"-> 0.007064131508  , \"τN\"-> 0.000028000819  , \"τC\"-> 0.006942241845  , \"κ0\"-> 0.000000023477  , \"T\"-> 3.000000000000  , \"mm1\"-> 0.000000000000  , \"mm2\"-> 0.000000000000  , \"mm3\"-> 0.000000000000  , \"θ\"-> 0.000000000000  |>   , \r61 ->   <| \"ζ\"-> 0.029251354442  , \"τ1\"-> 0.014634751206  , \"τS\"-> 0.003873958746  , \"τN\"-> 0.000007000487  , \"τC\"-> 0.006827504775  , \"κ0\"-> 0.000000056438  , \"T\"-> 5.500000000000  , \"mm1\"-> 0.000000000000  , \"mm2\"-> 0.000000000000  , \"mm3\"-> 0.000000000000  , \"θ\"-> 0.000000000000  |>   , \r70 ->   <| \"ζ\"-> 0.160286026344  , \"τ1\"-> 0.073452047785  , \"τS\"-> 0.044872374187  , \"τN\"-> 0.162076895387  , \"τC\"-> 0.001481759328  , \"κ0\"-> 0.000000001039  , \"T\"-> 0.179000000000  , \"mm1\"-> 0.000000000000  , \"mm2\"-> 0.000000000000  , \"mm3\"-> 0.000000000000  , \"θ\"-> 90.000000000000  |>   , \r71 ->   <| \"ζ\"-> 0.317192968490  , \"τ1\"-> 0.095324848000  , \"τS\"-> 0.087097785701  , \"τN\"-> 0.936221653169  , \"τC\"-> 0.001480807262  , \"κ0\"-> 0.000000000534  , \"T\"-> 0.120000000000  , \"mm1\"-> 0.000000000000  , \"mm2\"-> 0.000000000000  , \"mm3\"-> 0.000000000000  , \"θ\"-> 90.000000000000  |>   , \r72 ->   <| \"ζ\"-> 0.222764630124  , \"τ1\"-> 0.096058032825  , \"τS\"-> 0.066495942806  , \"τN\"-> 0.366151877245  , \"τC\"-> 0.001319275999  , \"κ0\"-> 0.000000000769  , \"T\"-> 0.148000000000  , \"mm1\"-> 0.000000000000  , \"mm2\"-> 0.000000000000  , \"mm3\"-> 0.000000000000  , \"θ\"-> 90.000000000000  |>   , \r73 ->   <| \"ζ\"-> 0.136082903087  , \"τ1\"-> 0.070214285183  , \"τS\"-> 0.041562366618  , \"τN\"-> 0.122478563978  , \"τC\"-> 0.001561716081  , \"κ0\"-> 0.000000001214  , \"T\"-> 0.197000000000  , \"mm1\"-> 0.000000000000  , \"mm2\"-> 0.000000000000  , \"mm3\"-> 0.000000000000  , \"θ\"-> 90.000000000000  |>   , \r74 ->   <| \"ζ\"-> 0.079924133870  , \"τ1\"-> 0.053892600038  , \"τS\"-> 0.033721986821  , \"τN\"-> 0.048194390820  , \"τC\"-> 0.001786420268  , \"κ0\"-> 0.000000001543  , \"T\"-> 0.249000000000  , \"mm1\"-> 0.000000000000  , \"mm2\"-> 0.000000000000  , \"mm3\"-> 0.000000000000  , \"θ\"-> 90.000000000000  |>   , \r75 ->   <| \"ζ\"-> 0.055680730504  , \"τ1\"-> 0.044845519236  , \"τS\"-> 0.029550773155  , \"τN\"-> 0.023428217313  , \"τC\"-> 0.002197475136  , \"κ0\"-> 0.000000001960  , \"T\"-> 0.300000000000  , \"mm1\"-> 0.000000000000  , \"mm2\"-> 0.000000000000  , \"mm3\"-> 0.000000000000  , \"θ\"-> 90.000000000000  |>   , \r76 ->   <| \"ζ\"-> 0.040648812263  , \"τ1\"-> 0.038083560479  , \"τS\"-> 0.026574795079  , \"τN\"-> 0.013361826633  , \"τC\"-> 0.002899405432  , \"κ0\"-> 0.000000002383  , \"T\"-> 0.360000000000  , \"mm1\"-> 0.000000000000  , \"mm2\"-> 0.000000000000  , \"mm3\"-> 0.000000000000  , \"θ\"-> 90.000000000000  |>   , \r77 ->   <| \"ζ\"-> 0.031873906103  , \"τ1\"-> 0.030223838950  , \"τS\"-> 0.024286132427  , \"τN\"-> 0.006926780152  , \"τC\"-> 0.002978043437  , \"κ0\"-> 0.000000002967  , \"T\"-> 0.430000000000  , \"mm1\"-> 0.000000000000  , \"mm2\"-> 0.000000000000  , \"mm3\"-> 0.000000000000  , \"θ\"-> 90.000000000000  |>   , \r78 ->   <| \"ζ\"-> 0.025948172116  , \"τ1\"-> 0.025051552712  , \"τS\"-> 0.022571188655  , \"τN\"-> 0.003812228812  , \"τC\"-> 0.003259730052  , \"κ0\"-> 0.000000003686  , \"T\"-> 0.512000000000  , \"mm1\"-> 0.000000000000  , \"mm2\"-> 0.000000000000  , \"mm3\"-> 0.000000000000  , \"θ\"-> 90.000000000000  |>   , \r79 ->   <| \"ζ\"-> 0.020946044060  , \"τ1\"-> 0.024756174566  , \"τS\"-> 0.021099556284  , \"τN\"-> 0.002276701384  , \"τC\"-> 0.004159440288  , \"κ0\"-> 0.000000004389  , \"T\"-> 0.610000000000  , \"mm1\"-> 0.000000000000  , \"mm2\"-> 0.000000000000  , \"mm3\"-> 0.000000000000  , \"θ\"-> 90.000000000000  |>   , \r80 ->   <| \"ζ\"-> 0.014774082145  , \"τ1\"-> 0.015773102766  , \"τS\"-> 0.018723894921  , \"τN\"-> 0.000790199963  , \"τC\"-> 0.005097561693  , \"κ0\"-> 0.000000006095  , \"T\"-> 0.810000000000  , \"mm1\"-> 0.000000000000  , \"mm2\"-> 0.000000000000  , \"mm3\"-> 0.000000000000  , \"θ\"-> 90.000000000000  |>   , \r81 ->   <| \"ζ\"-> 0.013971175207  , \"τ1\"-> 0.015831825440  , \"τS\"-> 0.017293056061  , \"τN\"-> 0.000406001835  , \"τC\"-> 0.005061653181  , \"κ0\"-> 0.000000008423  , \"T\"-> 1.100000000000  , \"mm1\"-> 0.000000000000  , \"mm2\"-> 0.000000000000  , \"mm3\"-> 0.000000000000  , \"θ\"-> 90.000000000000  |>   , \r82 ->   <| \"ζ\"-> 0.014703834330  , \"τ1\"-> 0.019025451961  , \"τS\"-> 0.011790469569  , \"τN\"-> 0.000107003492  , \"τC\"-> 0.007625608278  , \"κ0\"-> 0.000000014259  , \"T\"-> 1.800000000000  , \"mm1\"-> 0.000000000000  , \"mm2\"-> 0.000000000000  , \"mm3\"-> 0.000000000000  , \"θ\"-> 90.000000000000  |>   , \r83 ->   <| \"ζ\"-> 0.021950059397  , \"τ1\"-> 0.019029879523  , \"τS\"-> 0.006582834729  , \"τN\"-> 0.000028012011  , \"τC\"-> 0.009051896214  , \"κ0\"-> 0.000000024750  , \"T\"-> 3.000000000000  , \"mm1\"-> 0.000000000000  , \"mm2\"-> 0.000000000000  , \"mm3\"-> 0.000000000000  , \"θ\"-> 90.000000000000  |>   , \r84 ->   <| \"ζ\"-> 0.027897403691  , \"τ1\"-> 0.014639690770  , \"τS\"-> 0.004105291179  , \"τN\"-> 0.000006999171  , \"τC\"-> 0.007414449545  , \"κ0\"-> 0.000000059701  , \"T\"-> 5.700000000000  , \"mm1\"-> 0.000073450671  , \"mm2\"-> 0.014673310812  , \"mm3\"-> 0.011534391407  , \"θ\"-> 90.000000000000  |>   , \r"
  in  "input":enum32{"Page 1"}(tab)
  in  "String":string="\"T\"-> 8.200000,    \"ζ\"-> 0.003915  , \"τ1\"-> 0.009762  , \"τS\"-> 0.134375  , \"τN\"-> 0.000042  , \"τC\"-> 0.013647  , \"κ0\"-> 0.000000102341  , \"mm1\"-> 0.000048  , \"mm2\"-> 0.148545  , \"mm3\"-> 0.009759 "
  in  "parse! :p":bool
  in  "Read from file":path=path "/opt/new/Dropbox/desktop_data/Indium-nanocal-cell12-June2021/labview-ready-files/Indium_June2021_067_8.2K_35T_dc_sh_ark.dat"
  in  "load! :l":bool
  in  "backup string :b":string="\"T\"-> 0.225000,    \"ζ\"-> 0.006057  , \"τ1\"-> 0.011106  , \"τS\"-> 0.134857  , \"τN\"-> 0.000042  , \"τC\"-> 0.012982  , \"κ0\"-> 0.000000101776  , \"mm1\"-> 0.000071  , \"mm2\"-> 0.148631  , \"mm3\"-> 0.011103 "
  out "B (T)":dbl=35.0
  out "file index":i32=67
  out "T (K)":dbl=8.2 format="%#_10f"
  out "θ (deg)":dbl format="%#_10f"
  in  "plots":enum32{"Page 1", "Page 2"}(tab)
  out "Plot:  colors":cluster{"Freq out (Hz)":dbl[], dbl[]}[](graph)=[{"Freq out (Hz)"=[0.8, 1.0, 1.2, 1.2, 1.38, 1.4, 1.6, 1.83, 2.13, 2.55, 2.62, 2.74, 4.0, 8.2], [0.005139197614, 0.00503541695, 0.005025241341, 0.004777415229, 0.004568953302, 0.003888489419, 0.003310560377, 0.002815263504, 0.00286285388, 0.002469190413, 0.002412108852, 0.002669122108, 0.003123114807, 0.00391493831404709]}, {"Freq out (Hz)"=[0.8, 1.0, 1.2, 1.2, 1.38, 1.4, 1.6, 1.83, 2.13, 2.55, 2.62, 2.74, 4.0, 8.2], [0.198724796215, 0.122174929094, 0.102687516481, 0.096465030619, 0.093117776532, 0.0876011689, 0.073698198291, 0.065471361604, 0.054461176556, 0.040351968507, 0.040932774133, 0.038361259577, 0.020424162913, 0.009762017848695768]}, {"Freq out (Hz)"=[0.8, 1.0, 1.2, 1.2, 1.38, 1.4, 1.6, 1.83, 2.13, 2.55, 2.62, 2.74, 4.0, 8.2], [0.004800637014, 0.0062225146, 0.007383588614, 0.006885176015, 0.007355702079, 0.007032312731, 0.008858283837, 0.010801366154, 0.013607182187, 0.017885440476, 0.019260967968, 0.0211991111, 0.043527827747, 0.13437466196040418]}, {"Freq out (Hz)"=[0.8, 1.0, 1.2, 1.2, 1.38, 1.4, 1.6, 1.83, 2.13, 2.55, 2.62, 2.74, 4.0, 8.2], [0.465205171402, 0.205982547664, 0.103960168475, 0.081406405423, 0.062831572704, 0.055156103563, 0.033317244772, 0.021664996889, 0.011343205053, 0.005126718377, 0.005170470981, 0.003990494453, 0.000562268427, 4.235643214853134e-05]}, {"Freq out (Hz)"=[0.8, 1.0, 1.2, 1.2, 1.38, 1.4, 1.6, 1.83, 2.13, 2.55, 2.62, 2.74, 4.0, 8.2], [0.002863585191, 0.003366330966, 0.003866879432, 0.004205655089, 0.004650863735, 0.004551857108, 0.00548965562, 0.005770858189, 0.007225916211, 0.008463551777, 0.008253479704, 0.008668874028, 0.009966268738, 0.013647490503661961]}]
  in  "parameter selectors":enum32{"Page 1"}(tab)
  in  "select B (T)":u16(ring)=1 items=["12.000000"]
  in  "select θ (deg)":u16(ring) items=["0.000000", "90.000000"]
  in  "X selector":T2=enum."T(K)"
  in  "ignore T !":bool=TRUE
  in  "select T (T)":u16(ring) items=["0.120000", "0.148000", "0.179000", "0.197000", "0.249000", "0.250000", "0.300000", "0.360000", "0.430000", "0.512000", "0.610000", "0.810000", "1.100000", "1.120000", "1.800000", "3.000000", "5.500000", "5.700000"]
  in  "ignore B !":bool
  in  "ignore θ !":bool=TRUE
  in  "parameters":enum32{"Page 1"}(tab)
  in  "ζ":dbl(slide)=0.00391493831404709 min=0.0 max=0.3 step=1e-06 scale=1e-05..1000.0 scale format="%#_3p"
  in  "T1":dbl(slide)=0.009762017848695768 min=0.0 max=0.3 step=1e-06 scale=0.0001..10.0 scale format="%#_3p"
  in  "τS":dbl(slide)=0.13437466196040418 min=0.0 max=0.3 step=1e-06 scale=0.0001..10.0 scale format="%#_3p"
  in  "τN":dbl(slide)=4.235643214853134e-05 min=0.0 max=0.3 step=1e-06 scale=1e-06..10.0 scale format="%#_3p"
  in  "τC":dbl(slide)=0.013647490503661961 min=0.0 max=0.3 step=1e-06 scale=0.0001..10.0 scale format="%#_3p"
  in  "κ0":dbl(slide)=1.0234079529926423e-07 min=0.0 max=0.3 step=1e-12 scale=1e-10..1e-06 scale format="%#_3p"
  in  "newton control":enum32{"Page 1", "Page 2"}(tab)
  in  "pause! :":bool
  in  "newton control":enum32{"Page 1"}(tab)
  in  "# steps":dbl=250.0 format="%#_10f"
  in  "step":dbl(slide)=0.00011904714443717533 scale=1e-05..1.0 scale format="%#_3p"
  out "logarithmic derivatives":dbl[](array[numeric])=[0.05720491977594915, -4.516095325624162e-05, 0.007856704731282655, -0.0003054956692515763, -0.07623133012112922, -0.00011564211079189928]
  in  "what":cluster{"derivative":T2, "scaling":dbl}[](array[cluster])=[{"derivative"=enum."dζ", "scaling"=1.0}, {"derivative"=enum."dT1", "scaling"=1.0}, {"derivative"=enum."dτS", "scaling"=1.0}, {"derivative"=enum."dτN", "scaling"=1.0}, {"derivative"=enum."dτC", "scaling"=1.0}, {"derivative"=enum."dκ0", "scaling"=1.0}]
  in  "weighting":T3=enum."|dz/dω|"
  out "goodness":dbl=6.375258377440944e-05 format="%#_10f"
  in  "go! :":bool
  in  "newton pause":bool
  in  "sweeper panel":T4(tab)
  out "Plot: sweep window":cluster{"Freq out (Hz)":dbl[], dbl[]}[](graph)
  in  "scale gauge: Plot: complex plane":dbl(slide)=15384465.256376998 min=0.0 max=0.3 step=1e-06 scale=1e-05..100000000000.0 scale format="%#_3p"
  in  "ω0 (rad/sec)":dbl(slide)=140.85980015121274 scale=0.001..50000.0 scale format="%#_3f"
  in  "offset control tab":enum32{"Page 1"}(tab)
  in  "off\nRe\nIm":cluster{"Numeric":dbl, "Numeric":dbl}(slide)={"Numeric"=0.0, "Numeric"=-30864.197530864738} scale=-90000000.0..50000000.0 scale format="%#_1p"
  in  "cspan":dbl=0.003 format="%#_13g"
  in  "cursor window":T5={"left"=20184.313682072192, "right "=24669.14654231211, "center"=22426.730112192152, "window"=4484.832860239923, "cursors"=[0, 1, 2], "relative"=0, "absolute"=0, "fixed vertical offset"=0.0, "vertical offset"=0.0, "skew"=0.0, "default window frac"=0.1, "kind"=enum."symmetric", "skew.left"=0.5, "skew.right"=0.5, "Plot ref"=refnum, "wing order"=enum."forw"}
  in  "win":T6={"cen (Hz)"=23772.179970264126, "win (Hz)"=4484.832860239923, "left (Hz)"=21529.763540144166, "right (Hz)"=26014.596400384085}
  in  ":sweep is ON":bool
  in  "stopping criteria":T7={"function tolerance"=1e-06, "parameter tolerance"=1e-06, "max iterations"=100, "max function calls"=1000, "gradient tolerance"=1e-06, "max time (sec)"=-1.0}
  in  "uco! :u":bool
  in  "tr":enum16{"as is", "add - ω", "full rydh"}(ring)=enum."add - ω"
  out "Plot: phase":cluster{"Freq out (Hz)":dbl[], dbl[]}[](graph)
  in  "save data":enum32{"save/read"}(tab)
  in  "Save to file :s":bool
  in  "Freq sweep name template":T8={"prefix"="RuCl3-rod", "group"="f"}
  in  "Save folder":path=path "/opt/data"
  in  "freq sweep file name":string="f004_RuCl3-rod_060221.dat"
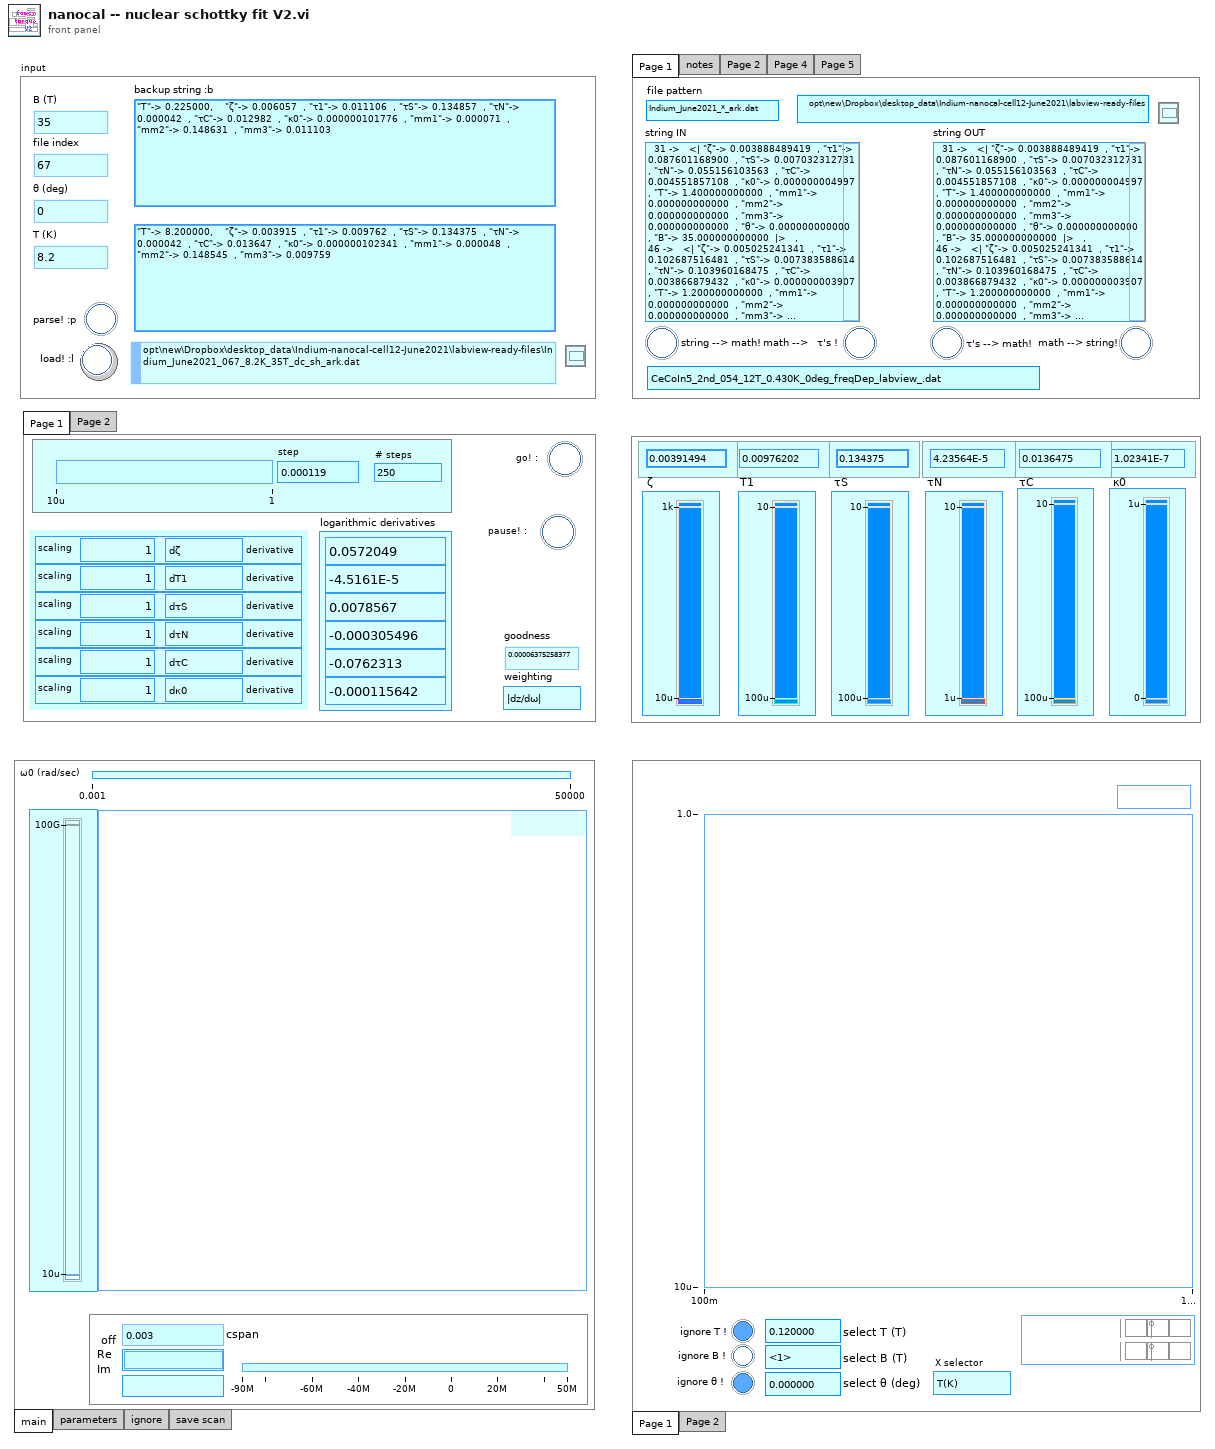
[diagram p1: front panel]
types:
  T1 = enum32{"Page 1", "notes", "Page 2", "Page 4", "Page 5"}
  T2 = typedef "3-lorentzian-heat-response action.ctl" = enum16{"calc R", "create string", "calc m1m2m3", "dζ", "dT1", "dτS", "dτN", "dτC", "d-all", "dκ0", "T(K)", "m1", "m2", "m3", "parse string", "θ (deg)", "B (T)"}
  T3 = typedef "nanocal-goodness-weighting-strategy.ctl" = enum16{"as is", "|dz/dω|", "ω", "phase"}
  T4 = enum32{"main", "parameters", "ignore", "save scan"}
  T5 = typedef "cursor winow.ctl" = cluster{"left":dbl, "right ":dbl, "center":dbl, "window":dbl, "cursors":i32[], "relative":i32, "absolute":i32, "fixed vertical offset":dbl, "vertical offset":dbl, "skew":dbl, "default window frac":dbl, "kind":enum16{"symmetric", "skewed", "fancy"}, "skew.left":dbl, "skew.right":dbl, "Plot ref":refnum<vi>, "wing order":enum16{"forw", "back"}}
  T6 = typedef "show-win- control.ctl" = cluster{"cen (Hz)":dbl, "win (Hz)":dbl, "left (Hz)":dbl, "right (Hz)":dbl}
  T7 = typedef "NI_Gmath.lvlib/stopping criteria.ctl" = cluster{"function tolerance":dbl, "parameter tolerance":dbl, "max iterations":i32, "max function calls":i32, "gradient tolerance":dbl, "max time (sec)":dbl}
  T8 = typedef "filename-pattern.ctl" = cluster{"prefix":string, "group":string}
  T9 = typedef "cursor action.ctl" = enum16{"range", "read", "write", "check", "zoom out", "smart zoom out", "zoom to aspect ratio 1", "zoom to win", "zoom out 20%", "zoom in 20%", "-empty", "smart zoom out&aspect", "move range left 20%", "move range right 20%", "move range up 20%", "move range down 20%", "zoom to X win", "zoom to Y win", "zoom out X", "zoom out Y", "zoom in X", "zoom in Y", "check plot scale"}
  T10 = typedef "cursor window action.ctl" = enum16{"balance", "h. offset change", "cursor moves", "change center", "change window", "init", "check", "reset", "set y to middle", "idle", "-write all Y", "-write left.X", "-write center.X", "-write right.X", "-write all X", "-change center", "-change window", "-change skew", "-read cursor 2", "-read cursor 1", "-read cursor 0", "-read all cursors", "-reset", "-read plot scale", "-set y to middle", "-Q: center.Y is visible", "-Q: window is visible", "-parse center.Y", "-right left from center", "-left move", "-right move", "-set center.Y", "-empty", "-set cursors to default", "-check", "-write center.Y", "-copy cursor 1", "-copy cursor 0", "-copy cursor 2", "move right", "move left", "shrink", "broaden", "skew up", "skew down", "-write plot scale", "zoom X", "change cen&win", "zoom to all data", "color--red", "color--green", "color--yellow", "read", "zoom out", "zoom in", "slide right", "slide left", "set range aspect ratio to 1"}
  T11 = typedef "publisher action.ctl" = enum16{"set", "get", "init", "check"}
  T12 = typedef "NI_Gmath.lvlib/objective function data.ctl" = variant
  T13 = typedef "filename-action.ctl" = enum16{"rewrite", "parse", "force pattern", "uniquenum", "get T", "get B", "get ind", "get deg", "get name", "get folder", "get extension", "get basename"}
  T14 = typedef "LVMapReplaceAction.ctl" = enum32{"Modify Entry only if found", "Add or Modify Entry", "Delete Entry"}
  T15 = typedef "file -- read-write control.ctl" = enum16{"read", "write all", "append one line"}
  T16 = typedef "array -- freq-voltage transformations action.ctl" = enum16{"as is", "add -ω", "sort ω", "2 x ω", "R-phase(deg) to Re-Im", "select ω>0"}
  T17 = typedef "KM_file -- read-write control.ctl" = enum16{"read", "write all", "append one line"}
  T18 = typedef "2Dwindow.ctl" = cluster{"window y":dbl, "center x":dbl, "center y":dbl, "window x":dbl}
  T19 = typedef "eventvkey.ctl" = enum16{"ASCII", "Enter", "Return", "Shift", "Ctrl", "Alt", "Cmd", "Opt", "Caps", "NumLock", "Clear", "Break", "Up", "Down", "Left", "Right", "Insert", "Delete", "Home", "End", "PageUp", "PageDown", "Escape", "Help", "Pause", "ScrollLock", "F1", "F2", "F3", "F4", "F5", "F6", "F7", "F8", "F9", "F10", "F11", "F12", "F13", "F14", "F15", "F16", "F17", "F18", "F19", "F20", "F21", "F22", "F23", "F24", "Play", "VolumeUp", "VolumeDown", "Mute", "Two Byte Char"}
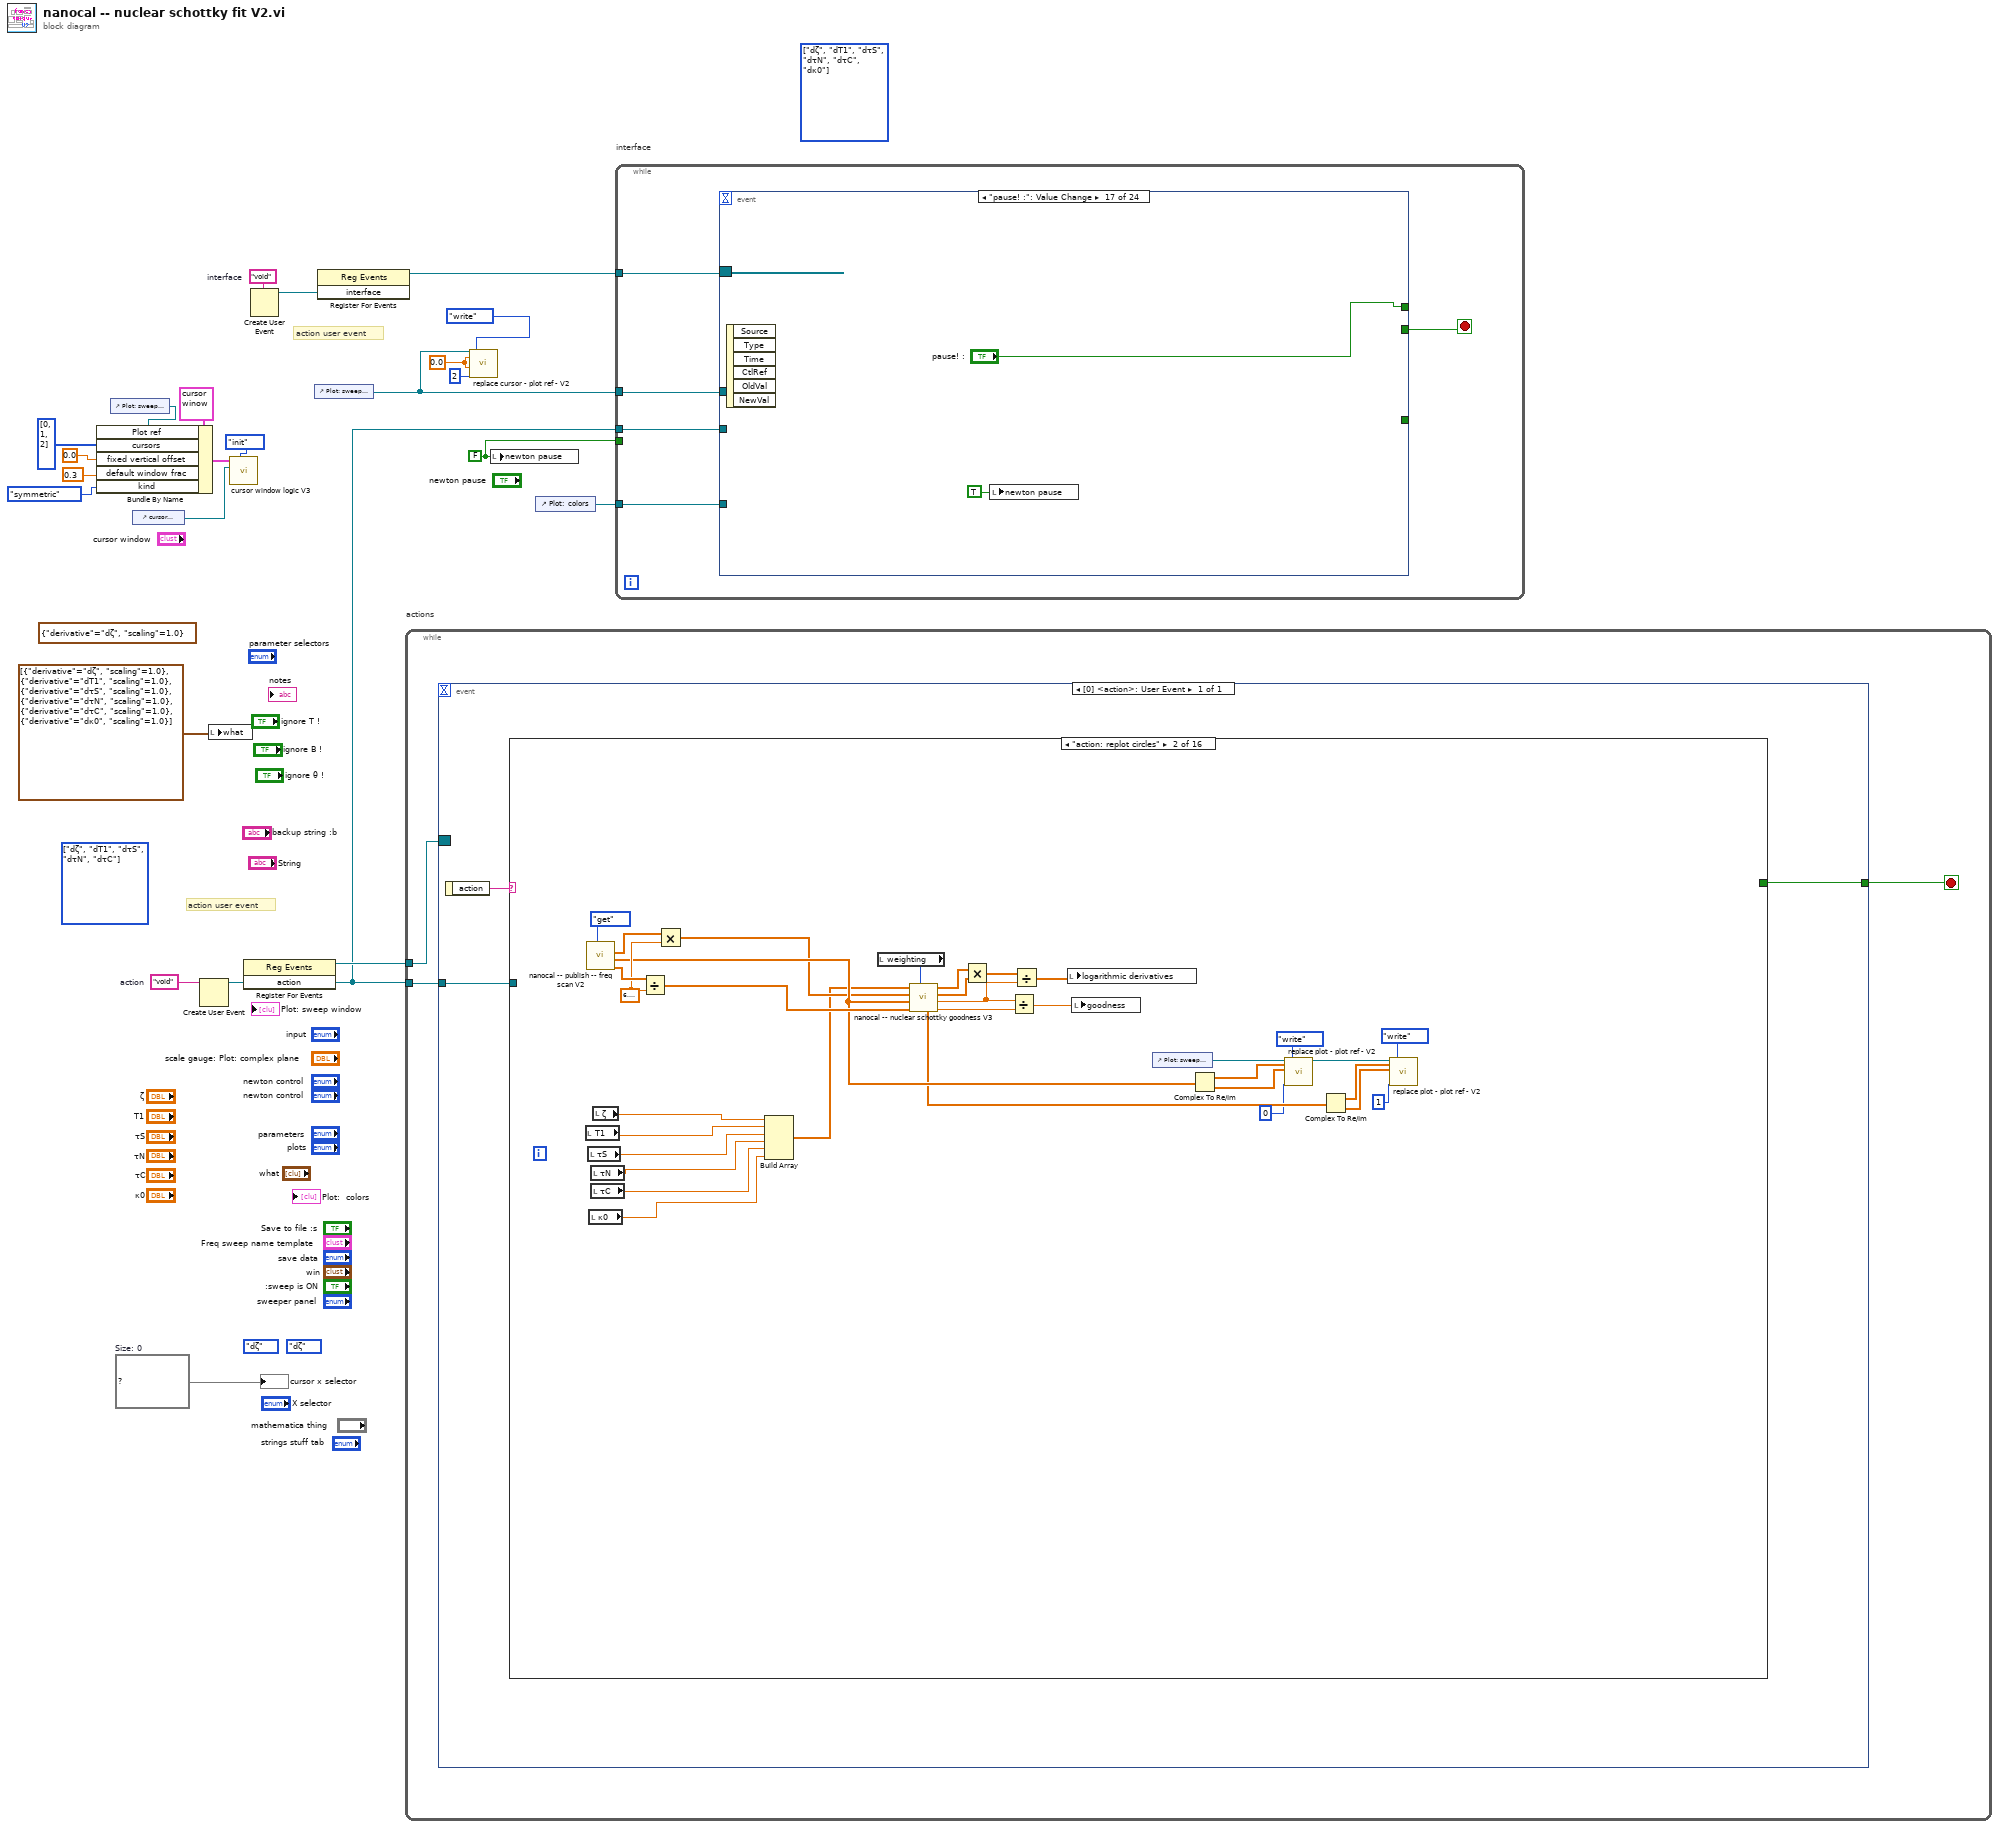
[diagram p0: block diagram]
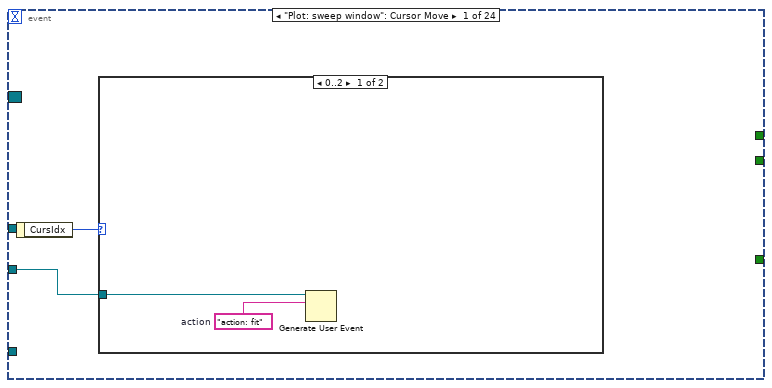
[diagram p2: hidden frame]
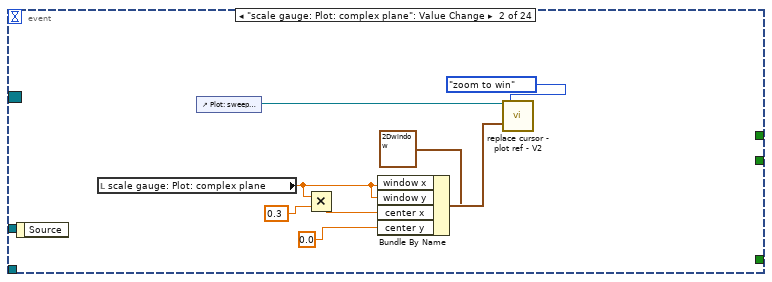
[diagram p4: hidden frame]
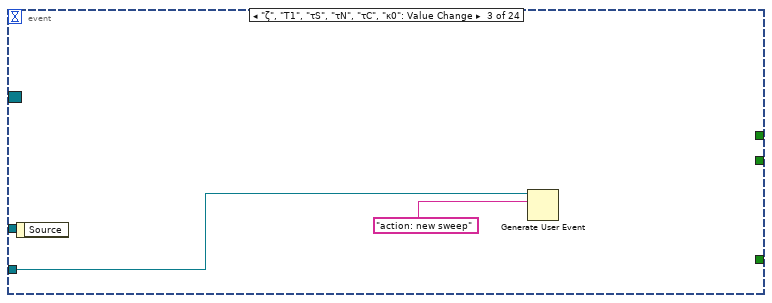
[diagram p5: hidden frame]
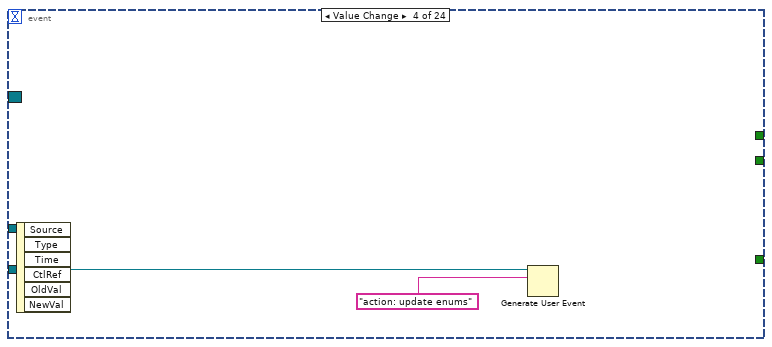
[diagram p6: hidden frame]
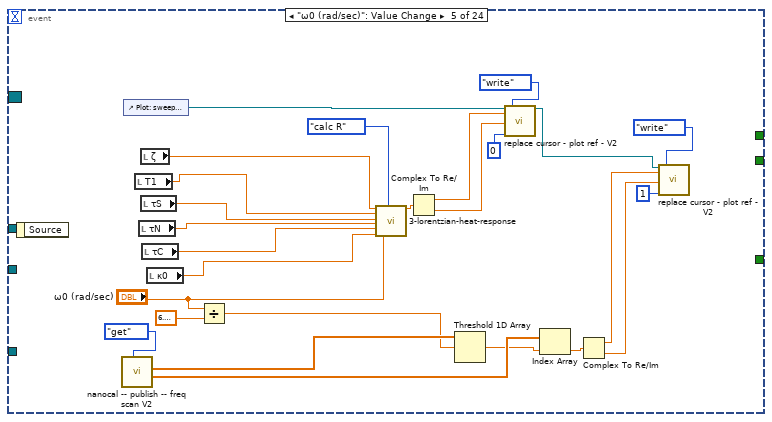
[diagram p7: hidden frame]
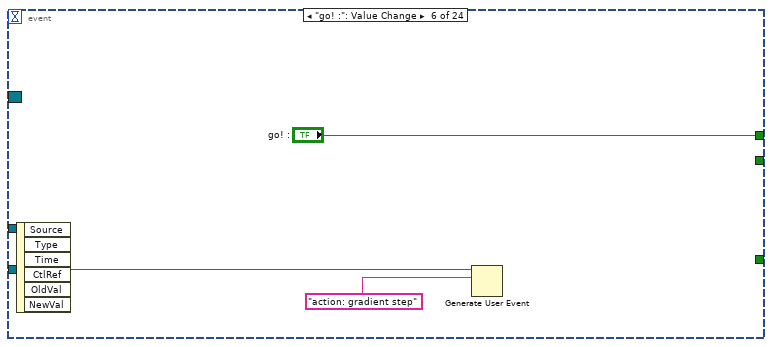
[diagram p8: hidden frame]
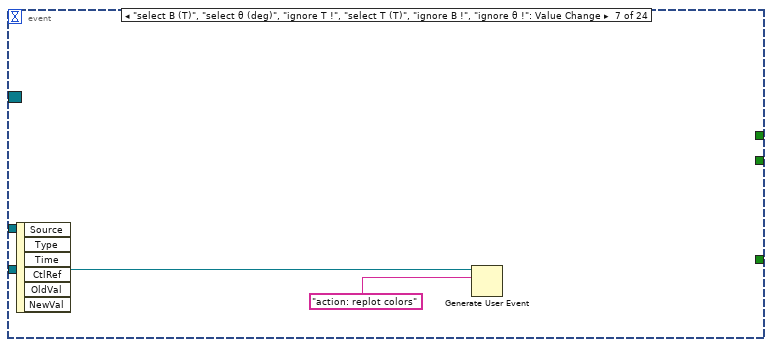
[diagram p9: hidden frame]
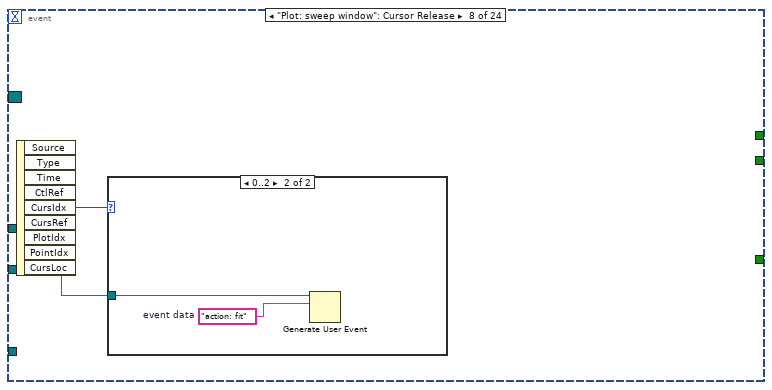
[diagram p10: hidden frame]
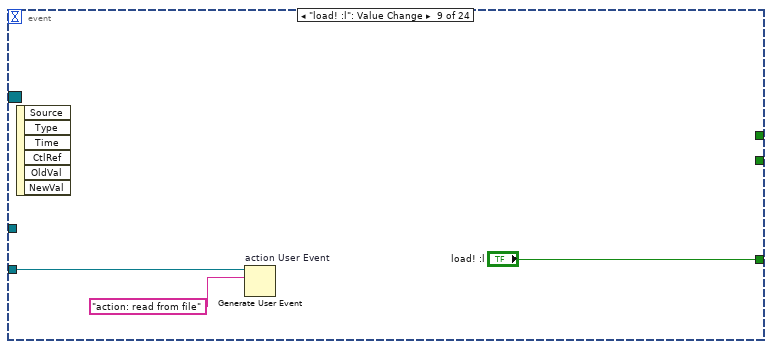
[diagram p12: hidden frame]
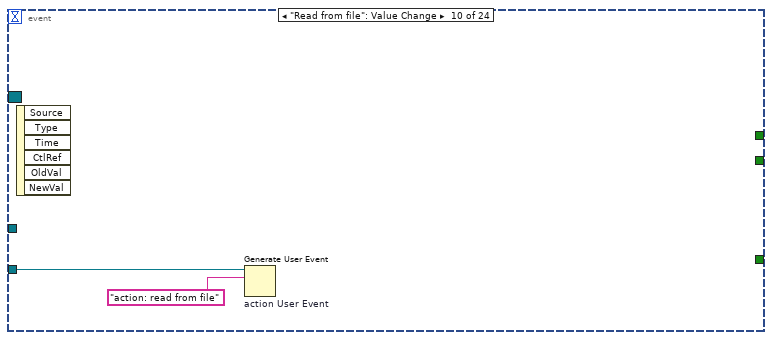
[diagram p13: hidden frame]
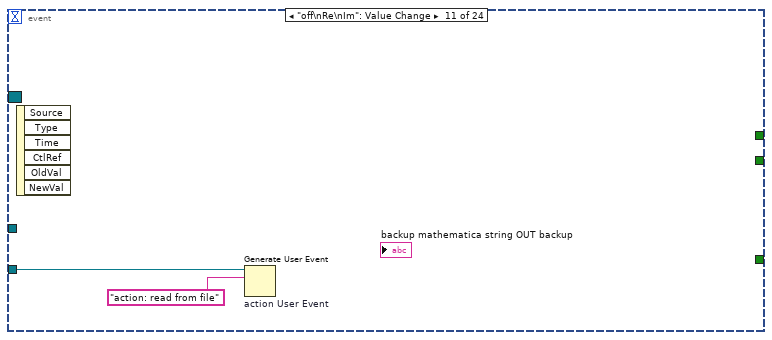
[diagram p14: hidden frame]
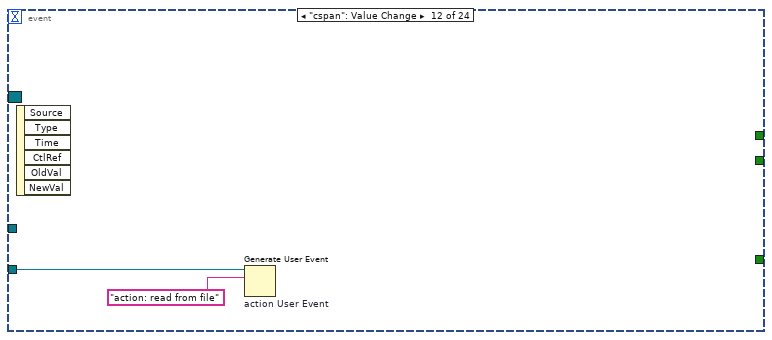
[diagram p15: hidden frame]
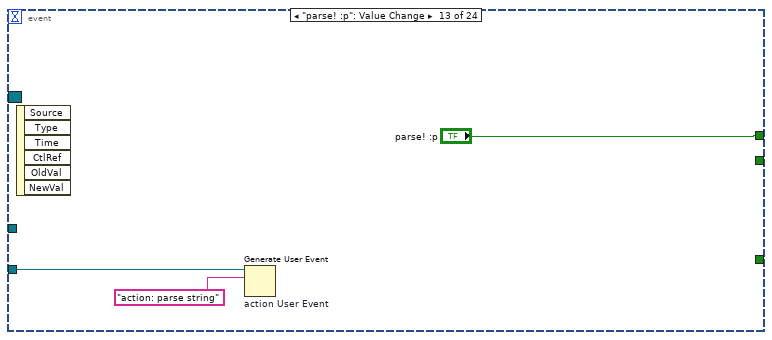
[diagram p16: hidden frame]
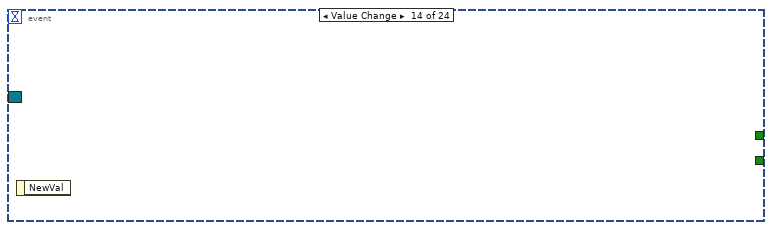
[diagram p17: hidden frame]
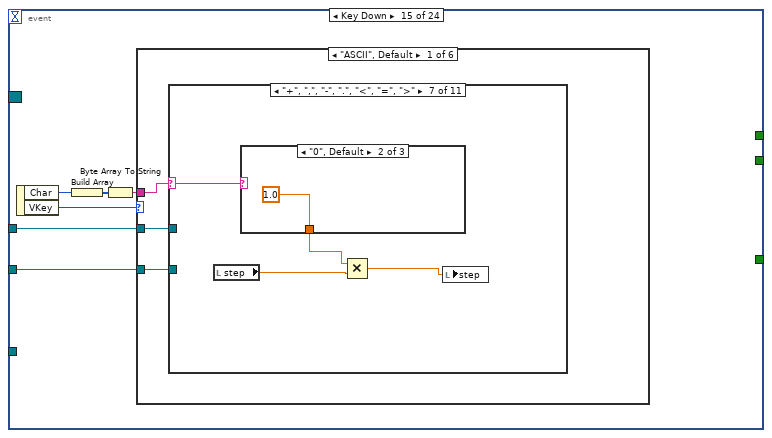
[diagram p18: hidden frame]
diagram:
  w1 = FALSE ("newton pause")
  (unwired) T2[] [enum."dζ", enum."dT1", enum."dτS", enum."dτN", enum."dτC", enum."dκ0"] items=["calc R", "create string", "calc m1m2m3", "dζ", "dT1", "dτS", "dτN", "dτC", "d-all", "dκ0", "T(K)", "m1", "m2", "m3", "parse string", "θ (deg)", "B (T)"] ("Array")
  w3 = map{T2, dbl} {}  # Size: 0
  (unwired) 3-lorentzian-heat-response_action."dζ" ("derivative")
  (unwired) 3-lorentzian-heat-response_action."dζ" ("derivative")
  w4 = 0.0 ("new X")
  (unwired) T2[] [enum."dζ", enum."dT1", enum."dτS", enum."dτN", enum."dτC"] items=["calc R", "create string", "calc m1m2m3", "dζ", "dT1", "dτS", "dτN", "dτC", "d-all", "dκ0", "T(K)", "m1", "m2", "m3", "parse string", "θ (deg)", "B (T)"] ("Array")
  (unwired) cluster{"derivative":T2, "scaling":dbl} {"derivative"=enum."dζ", "scaling"=1.0}
  w20 = "void"  # interface
  w22 = "void"  # action
  # "action user event"
  # "action user event"
  n1 = control-ref of="Plot: sweep window"() -> (w12:refnum<vi>)
  n2 = Bundle By Name(cluster=T5 {"left"=0.0, "right "=0.0, "center"=0.0, "window"=0.0, "cursors"=[], "relative"=0, "absolute"=0, "fixed vertical offset"=0.0, "vertical offset"=0.0, "skew"=0.0, "default window frac"=0.0, "kind"=enum."symmetric", "skew.left"=0.0, "skew.right"=0.0, "Plot ref"=refnum, "wing order"=enum."forw"} ("cursor bracket: All, data window"), "Plot ref"=w12, "cursors"=i32[] [0, 1, 2], "fixed vertical offset"=0.0, "default window frac"=0.3 ("fixed vertical offset"), "kind"=enum16{"symmetric", "skewed", "fancy"}."symmetric") -> (w15:T5)
  n3 = control-ref of="cursor window"() -> (w11:refnum<vi>)
  n4 = Create User Event(user event datatype=w22) -> (user event=w9:refnum<user-event>)  [unwired: 1 in, 1 out]
  n5 = local write "what"(cluster{"derivative":T2, "scaling":dbl}[] [{"derivative"=enum."dζ", "scaling"=1.0}, {"derivative"=enum."dT1", "scaling"=1.0}, {"derivative"=enum."dτS", "scaling"=1.0}, {"derivative"=enum."dτN", "scaling"=1.0}, {"derivative"=enum."dτC", "scaling"=1.0}, {"derivative"=enum."dκ0", "scaling"=1.0}]) -> ()
  n6 = call "cursor window logic V3.vi"("cursor window action"=cursor_window_action."init", "cursor window in"=w11, "cursor window init"=w15) -> ()  [unwired: 7 in, 2 out]
  n7 = register-events(w9) -> (reference out=w23:refnum<event-registration>)  [unwired: 2 in, 1 out]
  n8 = Create User Event(user event datatype=w20) -> (user event=w10:refnum<user-event>)  [unwired: 1 in, 1 out]
  n9 = control-ref of="Plot: sweep window"() -> (w5:refnum<vi>)
  n10 = register-events(w10) -> (reference out=w21:refnum<event-registration>)  [unwired: 2 in, 1 out]
  n11 = while "actions" {
    tunnel: w23 -> [w26]
    tunnel: w9 -> [w25]
    stop <- w24 stop-if-true
    n12 = event shown="[0] <action>: User Event" {
      selector: w26 -> [_]
      dyn-events: _ -> [_]
      timeout: _ -> [_]
      tunnel: w25 -> [w28]
      tunnel: [w27] -> w24
      event User Event {
        n13 = event-data() -> ("action"=w29:string)  [unwired: 1 in]
        n14 = case shown="\"action: replot circles\"" w29 {
          tunnel: w28 -> [_ _ w126 w225 w227 w249 w334 _ _ w462 w505 _ w554 _ _ _]
          tunnel: [_ _ _ _ _ _ _ _ _ _ _ TRUE _ _ _ _] -> w27
          frame "action: new sweep" {
            (unwired) cursor_action."write" ("cursor action")
            w72 = 6.283185307179586
            n15 = local read "T1"() -> (w43:dbl)
            n16 = call "nanocal -- publish -- freq scan V2.vi"("publisher action"=publisher_action."get") -> ("dz/dω out (V)"=w73:cdb[], "z out (V)"=w63:cdb[], "ω out (Hz)"=w75:dbl[])  [unwired: 8 in]
            n17 = local read "τS"() -> (w42:dbl)
            n18 = local read "κ0"() -> (w39:dbl)
            n19 = local read "τN"() -> (w41:dbl)
            n20 = local read "τC"() -> (w40:dbl)
            n21 = local read "ζ"() -> (w44:dbl)
            n22 = Divide(x=w73, y=w72) -> (x/y=w66:cdb[])
            n23 = Multiply(x=w75, y=w72) -> (x*y=w62:dbl[])
            n24 = Build Array(w44, w43, w42, w41, w40, w39) -> (w59:dbl[])
            n25 = local read "weighting"() -> (w65:T3)
            n26 = call "3-lorentzian-heat-response -- V3.vi"("action"=3-lorentzian-heat-response_action."calc m1m2m3", "parameters IN"=w59) -> ("m1m2m3 OUT"=w56:dbl[], "parameters OUT"=w57:dbl[])  [unwired: 5 in, 3 out]
            n27 = call "nanocal -- nuclear schottky goodness V3.vi"("weighting strategy"=w65, "dz/dω IN (V)"=w66, "Voltage IN (V)"=w63, "ω (rad/sec)"=w62, "parameters"=w59) -> ("R norm"=w54:dbl, "G"=w50:dbl, "derivatives"=w52:dbl[], "parameters OUT"=w53:dbl[], "R(ω) out"=w49:cdb[])  [unwired: 2 in]
            n28 = Multiply(x=w53, y=w52) -> (x*y=w51:dbl[])
            n29 = disable-structure shown="Disabled" {
              disable-tunnel: w63 -> [w84 _]
              disable-tunnel: w62 -> [w81 _]
              disable-tunnel: w49 -> [w77 _]
              frame Disabled {
                n30 = Complex To Polar(r * e^(i*theta)=w84) -> (theta=w83:dbl[])  [unwired: 1 out]
                n31 = Complex To Polar(r * e^(i*theta)=w77) -> (theta=w82:dbl[])  [unwired: 1 out]
                n32 = Bundle(w81, w83) -> (w80:cluster{dbl[], dbl[]})  [unwired: 1 in]
                n33 = Bundle(w81, w82) -> (w79:cluster{dbl[], dbl[]})  [unwired: 1 in]
                n34 = Build Array(w80, w79) -> (→"Plot: phase":cluster{dbl[], dbl[]}[])
                n35 = control-ref of="Plot: phase"() -> ()  [unwired: 1 out]
              }
              frame Enabled {
              }
            }
            n36 = Divide(x=w50, y=w54) -> (x/y=→"goodness":dbl)
            n37 = call "3-lorentzian-heat-response -- V3.vi"("action"=3-lorentzian-heat-response_action."create string", "m1m2m3 IN"=w56, "parameters IN"=w59) -> ("String out"=w58:string)  [unwired: 4 in, 4 out]
            n38 = local read "T (K)"() -> (w46:dbl)
            n39 = Divide(x=w51, y=w50) -> (x/y=→"logarithmic derivatives":dbl[])
            n40 = Build Array (concatenate)(w57, w56) -> (w55:dbl[])
            n41 = local read "cursor x selector"() -> (w48:map{T2, dbl})
            n42 = local read "X selector"() -> (w47:T2)
            n43 = Number To Fractional String(number=w46) -> (F-format string=w70:string)  [unwired: 3 in]
            n44 = control-ref of="Plot: sweep window"() -> (w38:refnum<vi>)
            n45 = Concatenate Strings("\"T\"-> ", w70, ",   ", w58) -> (w64:string)
            n46 = Look In Map(map=w48, key=w47, default value=w46) -> (value=w45:dbl)  [unwired: 1 out]
            n47 = control-ref of="Plot:  colors"() -> (w74:refnum<vi>)
            n48 = Complex To Re/Im(x + iy=w63) -> (x=w37:dbl[], y=w36:dbl[])
            n49 = local write "String"(w64) -> ()
            n50 = call "replace plot - plot ref - V2.vi"("Plot ref in"=w38, "Array X IN"=w37, "Array Y IN"=w36, "plot index"=0) -> ("Plot ref out"=w35:refnum<vi>)  [unwired: 12 in, 3 out]
            n51 = for {
              tunnel: w55 -> [w89] mode=indexing
              tunnel: w45 -> [w88]
              tunnel: w74 -> [w86]
              i -> [w85]
              n52 = call "replace cursor - plot ref - V2.vi"("Plot ref in"=w86, "new X"=w88, "new  Y"=w89, "cursor index"=w85, "cursor action"=cursor_action."write") -> ()  [unwired: 11 in, 4 out]
            }
            n53 = Complex To Re/Im(x + iy=w49) -> (x=w33:dbl[], y=w32:dbl[])
            n54 = call "replace plot - plot ref - V2.vi"("Plot ref in"=w35, "Array X IN"=w33, "Array Y IN"=w32, "plot index"=1, "cursor action"=cursor_action."write") -> ()  [unwired: 11 in, 4 out]
          }
          frame "action: replot circles" {
            w119 = 6.283185307179586
            n55 = local read "T1"() -> (w106:dbl)
            n56 = call "nanocal -- publish -- freq scan V2.vi"("publisher action"=publisher_action."get") -> ("dz/dω out (V)"=w120:cdb[], "z out (V)"=w116:cdb[], "ω out (Hz)"=w121:dbl[])  [unwired: 8 in]
            n57 = local read "τS"() -> (w105:dbl)
            n58 = local read "κ0"() -> (w102:dbl)
            n59 = local read "τN"() -> (w104:dbl)
            n60 = local read "τC"() -> (w103:dbl)
            n61 = local read "ζ"() -> (w107:dbl)
            n62 = Divide(x=w120, y=w119) -> (x/y=w118:cdb[])
            n63 = Multiply(x=w121, y=w119) -> (x*y=w115:dbl[])
            n64 = Build Array(w107, w106, w105, w104, w103, w102) -> (w114:dbl[])
            n65 = local read "weighting"() -> (w117:T3)
            n66 = call "nanocal -- nuclear schottky goodness V3.vi"("weighting strategy"=w117, "dz/dω IN (V)"=w118, "Voltage IN (V)"=w116, "ω (rad/sec)"=w115, "parameters"=w114) -> ("R norm"=w113:dbl, "G"=w109:dbl, "derivatives"=w111:dbl[], "parameters OUT"=w112:dbl[], "R(ω) out"=w108:cdb[])  [unwired: 2 in]
            n67 = Multiply(x=w112, y=w111) -> (x*y=w110:dbl[])
            n68 = Divide(x=w109, y=w113) -> (x/y=w100:dbl)
            n69 = Divide(x=w110, y=w109) -> (x/y=w101:dbl[])
            n70 = local write "logarithmic derivatives"(w101) -> ()
            n71 = local write "goodness"(w100) -> ()
            n72 = control-ref of="Plot: sweep window"() -> (w95:refnum<vi>)
            n73 = Complex To Re/Im(x + iy=w116) -> (x=w93:dbl[], y=w92:dbl[])
            n74 = call "replace plot - plot ref - V2.vi"("Plot ref in"=w95, "Array X IN"=w93, "Array Y IN"=w92, "plot index"=0, "cursor action"=cursor_action."write") -> ("Plot ref out"=w94:refnum<vi>)  [unwired: 11 in, 3 out]
            n75 = Complex To Re/Im(x + iy=w108) -> (x=w91:dbl[], y=w90:dbl[])
            n76 = call "replace plot - plot ref - V2.vi"("Plot ref in"=w94, "Array X IN"=w91, "Array Y IN"=w90, "plot index"=1, "cursor action"=cursor_action."write") -> ()  [unwired: 11 in, 4 out]
          }
          frame "action: gradient step" {
            w123 = FALSE ("newton pause")
            n77 = local write "newton pause"(w123) -> ()
            n78 = Generate User Event(user event=w126, event data cluster="action: new sweep" ("event data")) -> ()  [unwired: 2 in, 2 out]
            n79 = for {
              N: "# steps" -> [_]
              tunnel: [TRUE ("newton pause")] -> w124
              tunnel: w123 -> [_]
              stop <- w135 stop-if-true
              w160 = 6.283185307179586
              n80 = call "nanocal -- publish -- freq scan V2.vi"("publisher action"=publisher_action."get") -> ("dz/dω out (V)"=w161:cdb[], "z out (V)"=w175:cdb[], "ω out (Hz)"=w177:dbl[])  [unwired: 8 in]
              n81 = local read "newton pause"() -> (w135:bool)
              n82 = local read "T1"() -> (w151:dbl)
              n83 = local read "τS"() -> (w150:dbl)
              n84 = local read "τN"() -> (w149:dbl)
              n85 = local read "τC"() -> (w148:dbl)
              n86 = local read "κ0"() -> (w147:dbl)
              n87 = local read "ζ"() -> (w152:dbl)
              n88 = Divide(x=w161, y=w160) -> (x/y=w162:cdb[])
              n89 = Multiply(x=w177, y=w160) -> (x*y=w176:dbl[])
              n90 = local read "what"() -> (w179:cluster{"derivative":T2, "scaling":dbl}[])
              n91 = Build Array(w152, w151, w150, w149, w148, w147) -> (w145:dbl[])
              n92 = for {
                tunnel: w179 -> [w193] mode=indexing
                tunnel: [w192] -> w173 mode=indexing
                n93 = Unbundle By Name(w193) -> ("scaling"=w192:dbl)
              }
              n94 = call "nanocal -- nuclear schottky goodness V3.vi"("weighting strategy"="weighting", "dz/dω IN (V)"=w162, "Voltage IN (V)"=w175, "ω (rad/sec)"=w176, "parameters"=w145) -> ("R norm"=w144:dbl, "G"=w140:dbl, "derivatives"=w142:dbl[], "parameters OUT"=w143:dbl[], "R(ω) out"=w133:cdb[])  [unwired: 2 in]
              n95 = Multiply(x=w143, y=w142) -> (x*y=w141:dbl[])
              n96 = Divide(x=w140, y=w144) -> (x/y=w157:dbl)
              n97 = Divide(x=w141, y=w140) -> (x/y=w156:dbl[])
              n98 = Multiply(x=w173, y=w156) -> (x*y=w172:dbl[])
              n99 = Multiply(x=w172, y="step") -> (x*y=w182:dbl[])
              n100 = control-ref of="Plot: sweep window"() -> (w131:refnum<vi>)
              n101 = Subtract(x=1.0 ("index"), y=w182) -> (x-y=w170:dbl[])
              n102 = Complex To Re/Im(x + iy=w133) -> (x=w129:dbl[], y=w128:dbl[])
              n103 = Index Array(array=w170, index #1=0 ("index"), index #2=1 ("index"), index #3=2 ("index"), index #4=3 ("index"), index #5=4 ("index"), index #6=5 ("index")) -> (element #1=w171:dbl, element #2=w169:dbl, element #3=w168:dbl, element #4=w167:dbl, element #5=w166:dbl, element #6=w163:dbl)
              n104 = local read "cursor x selector"() -> (w139:map{T2, dbl})
              n105 = local read "X selector"() -> (w138:T2)
              n106 = local read "T (K)"() -> (w137:dbl)
              n107 = call "replace plot - plot ref - V2.vi"("Plot ref in"=w131, "Array X IN"=w129, "Array Y IN"=w128, "plot index"=1 ("index"), "cursor action"=cursor_action."write") -> ()  [unwired: 11 in, 4 out]
              n108 = local write "logarithmic derivatives"(w156) -> ()
              n109 = Multiply(x=w171, y=w152) -> (x*y=w187:dbl)
              n110 = Multiply(x=w169, y=w151) -> (x*y=w186:dbl)
              n111 = Multiply(x=w168, y=w150) -> (x*y=w185:dbl)
              n112 = local write "goodness"(w157) -> ()
              n113 = Multiply(x=w167, y=w149) -> (x*y=w184:dbl)
              n114 = control-ref of="Plot:  colors"() -> (w174:refnum<vi>)
              n115 = call "3-lorentzian-heat-response -- V3.vi"("action"=3-lorentzian-heat-response_action."calc m1m2m3", "parameters IN"=w145) -> ("m1m2m3 OUT"=w153:dbl[], "parameters OUT"=w154:dbl[])  [unwired: 5 in, 3 out]
              n116 = Look In Map(map=w139, key=w138, default value=w137) -> (value=w136:dbl)  [unwired: 1 out]
              n117 = Multiply(x=w166, y=w148) -> (x*y=w180:dbl)
              n118 = Build Array (concatenate)(w154, w153) -> (w146:dbl[])
              n119 = Multiply(x=w163, y=w147) -> (x*y=w165:dbl)
              n120 = local write "τN"(w184) -> ()
              n121 = local write "τC"(w180) -> ()
              n122 = local write "τS"(w185) -> ()
              n123 = local write "κ0"(w165) -> ()
              n124 = local write "T1"(w186) -> ()
              n125 = local write "ζ"(w187) -> ()
              n126 = for {
                tunnel: w146 -> [w198] mode=indexing
                tunnel: w136 -> [w197]
                tunnel: w174 -> [w195]
                i -> [w194]
                n127 = call "replace cursor - plot ref - V2.vi"("Plot ref in"=w195, "new X"=w197, "new  Y"=w198, "cursor index"=w194, "cursor action"=cursor_action."write") -> ()  [unwired: 11 in, 4 out]
              }
            }
            n128 = local write "newton pause"(w124) -> ()
          }
          frame "action: uco" {
            n129 = Generate User Event(user event=w225, event data cluster="action: new sweep" ("event data")) -> ()  [unwired: 2 in, 2 out]
            n130 = local read "T1"() -> (w217:dbl)
            n131 = local read "τS"() -> (w216:dbl)
            n132 = local read "τN"() -> (w215:dbl)
            n133 = local read "τC"() -> (w214:dbl)
            n134 = local read "κ0"() -> (w213:dbl)
            n135 = local read "ζ"() -> (w218:dbl)
            n136 = Build Array(w218, w217, w216, w215, w214, w213) -> (w205:dbl[])
            n137 = Natural Logarithm(1:w205) -> (0:w204:dbl[])
            n138 = vi-ref "nanocal -- nuclear schottky goodness -- for UCO -- V3.vi"() -> (w212:refnum<vi>)
            n139 = call-poly <vilib>:"Unconstrained Optimization.vi"("function data"=T12 variant, "objective function"=w212, "start"=w204) -> ("f(minimum)"=w201:dbl, "minimum"=w203:dbl[])  [unwired: 5 in, 2 out]
            n140 = Exponential(1:w201) -> (0:w200:dbl)
            n141 = Exponential(1:w203) -> (0:w202:dbl[])
            n142 = Index Array(array=w202, index #1=0 ("index"), index #2=1 ("index"), index #3=2 ("index"), index #4=3 ("index"), index #5=4 ("index"), index #6=5 ("index")) -> (element #1=w211:dbl, element #2=w210:dbl, element #3=w209:dbl, element #4=w208:dbl, element #5=w207:dbl, element #6=w206:dbl)
            n143 = local write "goodness"(w200) -> ()
            n144 = local write "τN"(w208) -> ()
            n145 = local write "τC"(w207) -> ()
            n146 = local write "τS"(w209) -> ()
            n147 = local write "κ0"(w206) -> ()
            n148 = local write "T1"(w210) -> ()
            n149 = local write "ζ"(w211) -> ()
          }
          frame "action: parse string" {
            w229 = T2[] [enum."dζ", enum."dT1", enum."dτS", enum."dτN", enum."dτC", enum."dκ0"] items=["calc R", "create string", "calc m1m2m3", "dζ", "dT1", "dτS", "dτN", "dτC", "d-all", "dκ0", "T(K)", "m1", "m2", "m3", "parse string", "θ (deg)", "B (T)"] ("Array")
            (unwired) 3-lorentzian-heat-response_action."dζ" ("derivative")
            n150 = local read "String"() -> (w244:string)
            n151 = call "string parse mathematica assosiated array.vi"("String in"=w244) -> ("Map"=w243:map{T2, dbl})  [unwired: 9 in, 1 out]
            n152 = Generate User Event "action User Event"(user event=w227, event data cluster="action: replot colors" ("event data")) -> ()  [unwired: 2 in, 2 out]
            n153 = for {
              tunnel: w243 -> [w247]
              tunnel: w229 -> [w246] mode=indexing
              tunnel: [w245] -> w236 mode=indexing
              n154 = Look In Map(map=w247, key=w246) -> (value=w245:dbl)  [unwired: 1 in, 1 out]
            }
            n155 = Index Array(array=w236, index #1=0 ("index"), index #2=1 ("index"), index #3=2 ("index"), index #4=3 ("index"), index #5=4 ("index"), index #6=5 ("index")) -> (element #1=w235:dbl, element #2=w234:dbl, element #3=w233:dbl, element #4=w232:dbl, element #5=w231:dbl, element #6=w230:dbl)
            n156 = local write "ζ"(w235) -> ()
            n157 = local write "T1"(w234) -> ()
            n158 = local write "τS"(w233) -> ()
            n159 = local write "τN"(w232) -> ()
            n160 = local write "τC"(w231) -> ()
            n161 = local write "κ0"(w230) -> ()
          }
          frame "action: read mathematica string" {
            w255 = map{T2, dbl} {}  # Size: 0
            w251 = set{dbl} {}  # Size: 0
            w258 = map{i32, map{T2, dbl}} {}  # Size: 0
            w259 = map{i32, string} {}  # Size: 0
            n162 = call "string parse mathematica list assosiated array.vi"("derivative"=3-lorentzian-heat-response_action."parse string", "string IN"="string IN") -> ("Map OUT"=w261:map{i32, map{T2, dbl}})  [unwired: 8 in, 1 out]
            n163 = List Folder(path="folder", pattern="file pattern") -> (filenames=w262:string[])  [unwired: 2 in, 3 out]
            n164 = Generate User Event(user event=w249, event data cluster="action: update enums" ("event data")) -> ()  [unwired: 2 in, 2 out]
            n165 = for {
              tunnel: w262 -> [w288] mode=indexing
              shift-right: [w293] -> w260
              shift-left: w261 -> [w295]
              shift-right: [w291] -> w256
              shift-left: w259 -> [w292]
              shift-right: [w266] -> w254
              shift-left: w258 -> [w267]
              shift-right: [w273] -> w252
              shift-left: w251 -> [w274]
              shift-right: [w276] -> w253
              shift-left: w251 -> [w277]
              tunnel: w255 -> [w282]
              shift-right: [w270] -> w248
              shift-left: w251 -> [w271]
              n166 = call "filename-manage.vi"("filename-action"=filename-action."get T", "file name IN"=w288) -> ("number OUT"=w272:dbl, "filename OUT"=w286:string)  [unwired: 7 in, 1 out]
              n167 = call "filename-manage.vi"("filename-action"=filename-action."get B", "file name IN"=w286) -> ("number OUT"=w278:dbl, "filename OUT"=w285:string)  [unwired: 7 in, 1 out]
              n168 = Insert Into Map(map in=w282, key=3-lorentzian-heat-response_action."T(K)", value=w272) -> (map out=w281:map{T2, dbl})  [unwired: 2 out]
              n169 = Insert Into Map(map in=w281, key=3-lorentzian-heat-response_action."B (T)", value=w278) -> (map out=w280:map{T2, dbl})  [unwired: 2 out]
              n170 = call "filename-manage.vi"("filename-action"=filename-action."get deg", "file name IN"=w285) -> ("number OUT"=w275:dbl, "filename OUT"=w299:string)  [unwired: 7 in, 1 out]
              n171 = Insert Into Map(map in=w280, key=3-lorentzian-heat-response_action."θ (deg)", value=w275) -> (map out=w269:map{T2, dbl})  [unwired: 2 out]
              n172 = call "filename-manage.vi"("filename-action"=filename-action."get ind", "file name IN"=w299) -> ("number OUT"=w294:dbl)  [unwired: 7 in, 2 out]
              n173 = To Long Integer(number=w294) -> (32bit integer=w268:i32)
              n174 = in-place {
                in-place-border: w278 -> [w333]
                in-place-border: w275 -> [w332]
                in-place-border: w272 -> [w323]
                in-place-border: [w322] -> w284
                n175 = in-place-map #1(w295, w268) -> (w326:map{T2, dbl}, w322:bool)  [unwired: 1 in]
                n176 = Insert Into Map(map in=w326, key=3-lorentzian-heat-response_action."T(K)", value=w323) -> (map out=w325:map{T2, dbl})  [unwired: 2 out]
                n177 = Insert Into Map(map in=w325, key=3-lorentzian-heat-response_action."B (T)", value=w333) -> (map out=w328:map{T2, dbl})  [unwired: 2 out]
                n178 = Insert Into Map(map in=w328, key=3-lorentzian-heat-response_action."θ (deg)", value=w332) -> (map out=w331:map{T2, dbl})  [unwired: 2 out]
                n179 = in-place-map #1(w331, LVMapReplaceAction."Modify Entry only if found" ("action")) -> (w293:map{i32, map{T2, dbl}})  [unwired: 2 out]
              }
              n180 = Not(x=w284) -> (.not. x?=w283:bool)
              n181 = case shown="True" w283 {
                tunnel: w292 -> [w304 w321]
                tunnel: [w304 w320] -> w291
                tunnel: w288 -> [_ w319]
                tunnel: w268 -> [_ w318]
                tunnel: w278 -> [_ w317]
                tunnel: w277 -> [w302 w316]
                tunnel: [w302 w315] -> w276
                tunnel: w275 -> [_ w314]
                tunnel: w274 -> [w303 w313]
                tunnel: [w303 w312] -> w273
                tunnel: w272 -> [_ w311]
                tunnel: [w300 w310] -> w270
                tunnel: w271 -> [w300 w309]
                tunnel: w269 -> [_ w308]
                tunnel: w268 -> [_ w307]
                tunnel: w267 -> [w301 w306]
                tunnel: [w301 w305] -> w266
                frame False {
                }
                frame True {
                  n182 = Insert Into Set(10:w311, 11:w309) -> (3:w310:set{dbl})  [unwired: 1 out]
                  n183 = Insert Into Set(10:w317, 11:w316) -> (3:w315:set{dbl})  [unwired: 1 out]
                  n184 = Insert Into Set(10:w314, 11:w313) -> (3:w312:set{dbl})  [unwired: 1 out]
                  n185 = Insert Into Map(map in=w306, key=w307, value=w308) -> (map out=w305:map{i32, map{T2, dbl}})  [unwired: 2 out]
                  n186 = Insert Into Map(map in=w321, key=w318, value=w319) -> (map out=w320:map{i32, string})  [unwired: 2 out]
                }
              }
            }
            "filenames" <- w256
            "temps&degs" <- w254
            "Set of B's" <- w253
            "Set of θ's" <- w252
            "Set of T's" <- w248
            n187 = local write "mathematica thing"(w260) -> ()
          }
          frame "action: update enums" {
            w339 = map{i32, dbl} {}  # Size: 0
            (unwired) set{dbl} {0.0, 5.0, 10.0, 15.0, 20.0, 25.0, 30.0, 35.0} ("Set of B's")
            (unwired) 3-lorentzian-heat-response_action."T(K)" ("key")
            w347 = map{i32, i32} {}  # Size: 0
            w346 = map{i32, dbl} {}  # Size: 0
            w345 = map{i32, dbl} {}  # Size: 0
            n188 = local read "temps&degs"() -> (w343:map{i32, map{T2, dbl}})
            n189 = local read "X selector"() -> (w342:T2)
            n190 = local read "filenames"() -> (w344:map{i32, string})
            n191 = Generate User Event(user event=w334, event data cluster="action: replot colors" ("event data")) -> ()  [unwired: 2 in, 2 out]
            n192 = for {
              tunnel: [w387] -> w354 mode=indexing
              tunnel: [w384] -> w352 mode=indexing
              tunnel: [w381] -> w356 mode=indexing
              tunnel: w342 -> [w385]
              tunnel: w344 -> [w383] mode=indexing
              tunnel: w343 -> [w382]
              n193 = Unbundle(w383) -> ("32bit integer"=w381:i32, "file pattern"=w387:string)
              n194 = Look In Map(map=w382, key=w381) -> (value=w386:map{T2, dbl})  [unwired: 1 in, 1 out]
              n195 = Look In Map(map=w386, key=w385) -> (value=w384:dbl)  [unwired: 1 in, 1 out]
            }
            n196 = call "array - sorted inexes.vi"("x"=w352) -> ("index array"=w353:i32[])  [unwired: 9 in, 1 out]
            n197 = local read "Set of T's"() -> (w338:set{dbl})
            n198 = local read "Set of B's"() -> (w340:set{dbl})
            n199 = local read "Set of θ's"() -> (w341:set{dbl})
            n200 = for {
              tunnel: w353 -> [w367] mode=indexing
              tunnel: w354 -> [w370]
              tunnel: [w369] -> w355 mode=indexing
              tunnel: w356 -> [w368]
              shift-right: [w363] -> w357
              shift-left: w347 -> [w366]
              i -> [w365]
              n201 = Index Array(array=w370, index=w367) -> (element=w369:string)
              n202 = Index Array(array=w368, index=w367) -> (element=w364:i32)
              n203 = Insert Into Map(map in=w366, key=w365, value=w364) -> (map out=w363:map{i32, i32})  [unwired: 2 out]
            }
            "filesnames lookup" <- w357
            n204 = for {
              shift-right: [w361] -> w337
              shift-left: w339 -> [w362]
              tunnel: [w359] -> w336 mode=indexing
              tunnel: w338 -> [w358] mode=indexing
              i -> [w360]
              n205 = Insert Into Map(map in=w362, key=w360, value=w358) -> (map out=w361:map{i32, dbl})  [unwired: 2 out]
              n206 = Number To Fractional String(number=w358) -> (F-format string=w359:string)  [unwired: 3 in]
            }
            "T lookup" <- w337
            n207 = for {
              shift-right: [w374] -> w351
              shift-left: w346 -> [w375]
              tunnel: [w372] -> w350 mode=indexing
              tunnel: w340 -> [w371] mode=indexing
              i -> [w373]
              n208 = Insert Into Map(map in=w375, key=w373, value=w371) -> (map out=w374:map{i32, dbl})  [unwired: 2 out]
              n209 = Number To Fractional String(number=w371) -> (F-format string=w372:string)  [unwired: 3 in]
            }
            "B lookup" <- w351
            n210 = for {
              shift-right: [w379] -> w349
              shift-left: w345 -> [w380]
              tunnel: [w377] -> w348 mode=indexing
              tunnel: w341 -> [w376] mode=indexing
              i -> [w378]
              n211 = Insert Into Map(map in=w380, key=w378, value=w376) -> (map out=w379:map{i32, dbl})  [unwired: 2 out]
              n212 = Number To Fractional String(number=w376) -> (F-format string=w377:string)  [unwired: 3 in]
            }
            "θ lookup" <- w349
            n213 = property on="select T (T)" class="Ring (strict)"("Strings []"=w336) -> ()  [unwired: 2 in, 2 out]
            n214 = property on="select B (T)" class="Ring (strict)"("Strings []"=w350) -> ()  [unwired: 2 in, 2 out]
            n215 = property on="select θ (deg)" class="Ring (strict)"("Strings []"=w348) -> ()  [unwired: 2 in, 2 out]
            n216 = property on="filenames" class="Ring (strict)"("Strings []"=w355) -> ()  [unwired: 2 in, 2 out]
          }
          frame "action: write mathematica string" {
            n217 = local read "mathematica thing"() -> (w389:map{i32, map{T2, dbl}})
            n218 = call "string parse mathematica list assosiated array.vi"("derivative"=3-lorentzian-heat-response_action."create string", "Map IN"=w389) -> ("string out"=→"string OUT":string)  [unwired: 8 in, 1 out]
          }
          frame "action: replot colors" {
            (unwired) 3-lorentzian-heat-response_action."T(K)" ("key")
            w408 = T2[] [enum."dζ", enum."dT1", enum."dτS", enum."dτN", enum."dτC"] items=["calc R", "create string", "calc m1m2m3", "dζ", "dT1", "dτS", "dτN", "dτC", "d-all", "dκ0", "T(K)", "m1", "m2", "m3", "parse string", "θ (deg)", "B (T)"] ("Array")
            n219 = local read "mathematica thing"() -> (w407:map{i32, map{T2, dbl}})
            n220 = local read "select θ (deg)"() -> (w405:u16)
            n221 = local read "ignore T !"() -> (w394:bool)
            n222 = local read "select B (T)"() -> (w400:u16)
            n223 = local read "select T (T)"() -> (w397:u16)
            n224 = local read "ignore B !"() -> (w393:bool)
            n225 = local read "θ lookup"() -> (w406:map{i32, dbl})
            n226 = local read "ignore θ !"() -> (w392:bool)
            n227 = local read "X selector"() -> (w391:T2)
            n228 = local read "T lookup"() -> (w398:map{i32, dbl})
            n229 = local read "B lookup"() -> (w401:map{i32, dbl})
            n230 = Look In Map(map=w398, key=w397) -> (value=w395:dbl)  [unwired: 1 in, 1 out]
            n231 = Look In Map(map=w406, key=w405) -> (value=w404:dbl)  [unwired: 1 in, 1 out]
            n232 = Look In Map(map=w401, key=w400) -> (value=w399:dbl)  [unwired: 1 in, 1 out]
            n233 = for {
              tunnel: w407 -> [w429]
              tunnel: w408 -> [w428] mode=indexing
              tunnel: w404 -> [w424]
              tunnel: 3-lorentzian-heat-response_action."θ (deg)" ("key") -> [w423]
              tunnel: w391 -> [w422]
              tunnel: 3-lorentzian-heat-response_action."B (T)" ("key") -> [w421]
              tunnel: w399 -> [w420]
              tunnel: 3-lorentzian-heat-response_action."T(K)" ("derivative") -> [w419]
              tunnel: w395 -> [w418]
              tunnel: w394 -> [w417]
              tunnel: w393 -> [w416]
              tunnel: w392 -> [w415]
              i -> [w412]
              n234 = for {
                tunnel: w429 -> [w461] mode=indexing
                tunnel: w428 -> [w460]
                tunnel: [w459] -> w427 mode=indexing if=w436
                tunnel: [w458] -> w426 mode=indexing if=w436
                tunnel: w424 -> [w456]
                tunnel: w423 -> [w455]
                tunnel: w422 -> [w454]
                tunnel: w421 -> [w452]
                tunnel: w420 -> [w451]
                tunnel: w419 -> [w449]
                tunnel: w418 -> [w440]
                tunnel: w417 -> [w439]
                tunnel: w416 -> [w448]
                tunnel: w415 -> [w446]
                tunnel: [w444] -> w414 mode=indexing if=w436
                n235 = Unbundle(w461) -> ("index"=w444:i32, "Map"=w450:map{T2, dbl})
                n236 = Look In Map(map=w450, key=w452) -> (value=w453:dbl)  [unwired: 1 in, 1 out]
                n237 = Look In Map(map=w450, key=w454) -> (value=w459:dbl)  [unwired: 1 in, 1 out]
                n238 = Look In Map(map=w450, key=w455) -> (value=w457:dbl)  [unwired: 1 in, 1 out]
                n239 = Look In Map(map=w450, key=w460) -> (value=w458:dbl)  [unwired: 1 in, 1 out]
                n240 = Look In Map(map=w450, key=w449) -> (value=w441:dbl)  [unwired: 1 in, 1 out]
                n241 = Equal?(x=w453, y=w451) -> (x = y?=w447:bool)
                n242 = Equal?(x=w441, y=w440) -> (x = y?=w438:bool)
                n243 = Equal?(x=w457, y=w456) -> (x = y?=w445:bool)
                n244 = Or(x=w439, y=w438) -> (x .or. y?=w437:bool)
                n245 = Or(x=w448, y=w447) -> (x .or. y?=w443:bool)
                n246 = Or(x=w446, y=w445) -> (x .or. y?=w442:bool)
                n247 = Compound Arithmetic op=AND(w437, w443, w442) -> (w436:bool)
              }
              n248 = call "array - sorted inexes.vi"("x"=w427) -> ("index array"=w425:i32[])  [unwired: 9 in, 1 out]
              n249 = for {
                tunnel: w427 -> [w435]
                tunnel: w426 -> [w434]
                tunnel: w425 -> [w430] mode=indexing
                tunnel: [w433] -> w411 mode=indexing
                tunnel: [w432] -> w410 mode=indexing
                tunnel: w414 -> [w431]
                n250 = Index Array(array=w431, index=w430) -> ()  [unwired: 1 out]
                n251 = Index Array(array=w435, index=w430) -> (element=w433:dbl)
                n252 = Index Array(array=w434, index=w430) -> (element=w432:dbl)
              }
              n253 = control-ref of="Plot:  colors"() -> (w409:refnum<vi>)
              n254 = call "replace plot - plot ref - V2.vi"("Plot ref in"=w409, "Array X IN"=w411, "Array Y IN"=w410, "plot index"=w412, "cursor action"=cursor_action."write") -> ()  [unwired: 11 in, 4 out]
            }
          }
          frame "action: copy from math" {
            w468 = T2[] [enum."dζ", enum."dT1", enum."dτS", enum."dτN", enum."dτC", enum."dκ0"] items=["calc R", "create string", "calc m1m2m3", "dζ", "dT1", "dτS", "dτN", "dτC", "d-all", "dκ0", "T(K)", "m1", "m2", "m3", "parse string", "θ (deg)", "B (T)"] ("Array")
            (unwired) 3-lorentzian-heat-response_action."dζ" ("derivative")
            n255 = local read "mathematica thing"() -> (w467:map{i32, map{T2, dbl}})
            n256 = local read "file index"() -> (w466:i32)
            n257 = Look In Map(map=w467, key=w466) -> (key not found?=w464:bool, value=w465:map{T2, dbl})  [unwired: 1 in]
            n258 = Generate User Event(user event=w462, event data cluster="action: new sweep" ("event data")) -> ()  [unwired: 2 in, 2 out]
            n259 = case shown="False" w464 {
              tunnel: w468 -> [w470 _]
              tunnel: w465 -> [w469 _]
              frame False {
                n260 = for {
                  tunnel: w469 -> [w486]
                  tunnel: w470 -> [w485] mode=indexing
                  tunnel: [w484] -> w477 mode=indexing
                  n261 = Look In Map(map=w486, key=w485) -> (value=w484:dbl)  [unwired: 1 in, 1 out]
                }
                n262 = Index Array(array=w477, index #1=0 ("index"), index #2=1 ("index"), index #3=2 ("index"), index #4=3 ("index"), index #5=4 ("index"), index #6=5 ("index")) -> (element #1=w476:dbl, element #2=w475:dbl, element #3=w474:dbl, element #4=w473:dbl, element #5=w472:dbl, element #6=w471:dbl)
                n263 = local write "ζ"(w476) -> ()
                n264 = local write "T1"(w475) -> ()
                n265 = local write "τS"(w474) -> ()
                n266 = local write "τN"(w473) -> ()
                n267 = local write "τC"(w472) -> ()
                n268 = local write "κ0"(w471) -> ()
              }
              frame True {
              }
            }
          }
          frame "action: copy to math" {
            w496 = T2[] [enum."dζ", enum."dT1", enum."dτS", enum."dτN", enum."dτC", enum."dκ0", enum."m1", enum."m2", enum."m3", enum."T(K)", enum."θ (deg)", enum."B (T)"] items=["calc R", "create string", "calc m1m2m3", "dζ", "dT1", "dτS", "dτN", "dτC", "d-all", "dκ0", "T(K)", "m1", "m2", "m3", "parse string", "θ (deg)", "B (T)"] ("Array")
            (unwired) 3-lorentzian-heat-response_action."dζ" ("derivative")
            n269 = local read "θ (deg)"() -> (w488:dbl)
            n270 = local read "B (T)"() -> (w487:dbl)
            n271 = local read "T (K)"() -> (w489:dbl)
            n272 = local read "ζ"() -> (w504:dbl)
            n273 = local read "T1"() -> (w503:dbl)
            n274 = local read "τS"() -> (w502:dbl)
            n275 = local read "τN"() -> (w501:dbl)
            n276 = local read "τC"() -> (w500:dbl)
            n277 = local read "κ0"() -> (w499:dbl)
            n278 = Build Array(w504, w503, w502, w501, w500, w499) -> (w492:dbl[])
            n279 = local read "mathematica thing"() -> (w498:map{i32, map{T2, dbl}})
            n280 = local read "file index"() -> (w497:i32)
            n281 = call "3-lorentzian-heat-response -- V3.vi"("action"=3-lorentzian-heat-response_action."calc m1m2m3", "parameters IN"=w492) -> ("m1m2m3 OUT"=w493:dbl[], "parameters OUT"=w494:dbl[])  [unwired: 5 in, 3 out]
            n282 = Build Array (concatenate)(w494, w493, w489, w488, w487) -> (w490:dbl[])
            n283 = in-place {
              in-place-border: w496 -> [w511]
              in-place-border: w490 -> [w507]
              n284 = in-place-map #2(w498, w497) -> (w510:map{T2, dbl})  [unwired: 1 in, 1 out]
              n285 = for {
                tunnel: w511 -> [w513] mode=indexing
                shift-right: [w514] -> w509
                shift-left: w510 -> [w515]
                tunnel: w507 -> [w512] mode=indexing
                n286 = Insert Into Map(map in=w515, key=w513, value=w512) -> (map out=w514:map{T2, dbl})  [unwired: 2 out]
              }
              n287 = in-place-map #2(w509, LVMapReplaceAction."Modify Entry only if found" ("action")) -> (w491:map{i32, map{T2, dbl}})  [unwired: 2 out]
            }
            n288 = Generate User Event(user event=w505, event data cluster="action: replot colors" ("event data")) -> ()  [unwired: 2 in, 2 out]
            n289 = local write "mathematica thing"(w491) -> ()
          }
          frame "action: exit" {
          }
          frame "action: read from file" {
            n290 = call "file - read-write - list of lines.vi"("read/write control"=file_--_read-write_control."read", "file path"="Read from file") -> ("list of lines OUT"=w557:string[], "filename out"=w550:string)  [unwired: 7 in, 1 out]
            n291 = local read "cursor x selector"() -> (w526:map{T2, dbl})
            n292 = for {
              tunnel: w557 -> [w591] mode=indexing
              tunnel: [w586] -> w534 mode=indexing if=w582
              tunnel: [w585] -> w553 mode=indexing if=w582
              w587 = 0.0
              n293 = Scan From String(format string="%f%f%f", input string=w591, initial scan location=u32 0, default 1=w587, default 2=w587, default 3=w587) -> (offset past scan=w583:u32, output 1=w585:dbl, output 2=w589:dbl, output 3=w588:dbl)  [unwired: 1 in, 2 out]
              n294 = Greater Than 0?(x=w583) -> (x > 0?=w582:bool)
              n295 = Re/Im To Complex(1:w588, 2:w589) -> (0:w586:cdb)
            }
            n296 = call "filename-manage.vi"("filename-action"=filename-action."get name", "file name IN"=w550) -> ("string OUT"=w547:string)  [unwired: 7 in, 2 out]
            n297 = call "filename-manage.vi"("filename-action"=filename-action."get T", "file name IN"=w547) -> ("number OUT"=w524:dbl, "filename OUT"=w546:string)  [unwired: 7 in, 1 out]
            "T (K)" <- w524
            n298 = Unbundle("off\nRe\nIm") -> ("Numeric"=w530:dbl, "Numeric"=w529:dbl)
            n299 = Re/Im To Complex(1:w529, 2:w530) -> (0:w533:cdb)
            n300 = Insert Into Map(map in=w526, key=3-lorentzian-heat-response_action."T(K)" ("derivative"), value=w524) -> (map out=w523:map{T2, dbl})  [unwired: 2 out]
            n301 = Subtract(x=w534, y=w533) -> (x-y=w532:cdb[])
            n302 = call "filename-manage.vi"("filename-action"=filename-action."get deg", "file name IN"=w546) -> ("number OUT"=w519:dbl, "filename OUT"=w536:string)  [unwired: 7 in, 1 out]
            "θ (deg)" <- w519
            n303 = Generate User Event(user event=w554, event data cluster="action: new sweep" ("event data")) -> ()  [unwired: 2 in, 2 out]
            n304 = case shown="\"add - ω\"" "tr" {
              tunnel: w532 -> [w558 w560 w572]
              tunnel: w553 -> [w559 w567 w581]
              tunnel: [w559 w564 w578] -> w543
              tunnel: [w558 w563 w577] -> w535
              frame "as is", Default {
              }
              frame "add - ω" {
                n305 = call "array -- freq-voltage transformations.vi"("freq voltage action"=array_--_freq-voltage_transformations_action."add -ω", "z In"=w560, "ω IN"=w567) -> ("z out"=w565:cdb[], "ω out"=w566:dbl[])  [unwired: 7 in]
                n306 = call "array -- freq-voltage transformations.vi"("freq voltage action"=array_--_freq-voltage_transformations_action."sort ω", "z In"=w565, "ω IN"=w566) -> ("z out"=w563:cdb[], "ω out"=w564:dbl[])  [unwired: 7 in]
              }
              frame "full rydh" {
                n307 = call "array -- freq-voltage transformations.vi"("freq voltage action"=array_--_freq-voltage_transformations_action."2 x ω", "z In"=w572, "ω IN"=w581) -> ("z out"=w571:cdb[], "ω out"=w574:dbl[])  [unwired: 7 in]
                n308 = call "array -- freq-voltage transformations.vi"("freq voltage action"=array_--_freq-voltage_transformations_action."R-phase(deg) to Re-Im", "z In"=w571, "ω IN"=w574) -> ("z out"=w570:cdb[], "ω out"=w573:dbl[])  [unwired: 7 in]
                n309 = call "array -- freq-voltage transformations.vi"("freq voltage action"=array_--_freq-voltage_transformations_action."add -ω", "z In"=w570, "ω IN"=w573) -> ("z out"=w579:cdb[], "ω out"=w580:dbl[])  [unwired: 7 in]
                n310 = call "array -- freq-voltage transformations.vi"("freq voltage action"=array_--_freq-voltage_transformations_action."sort ω", "z In"=w579, "ω IN"=w580) -> ("z out"=w577:cdb[], "ω out"=w578:dbl[])  [unwired: 7 in]
              }
            }
            n311 = Insert Into Map(map in=w523, key=3-lorentzian-heat-response_action."θ (deg)" ("derivative"), value=w519) -> (map out=w522:map{T2, dbl})  [unwired: 2 out]
            n312 = call "filename-manage.vi"("filename-action"=filename-action."get ind", "file name IN"=w536) -> ("number OUT"=→"file index":dbl, "filename OUT"=w528:string)  [unwired: 7 in, 1 out]
            n313 = call "filename-manage.vi"("filename-action"=filename-action."get B", "file name IN"=w528) -> ("number OUT"=w517:dbl)  [unwired: 7 in, 2 out]
            "B (T)" <- w517
            n314 = Insert Into Map(map in=w522, key=3-lorentzian-heat-response_action."B (T)" ("derivative"), value=w517) -> (map out=w521:map{T2, dbl})  [unwired: 2 out]
            n315 = call "filter - complex - four.vi"("omega  in"=w543, "z in"=w535, "span"="cspan") -> ("omega out"=w542:dbl[], "z out"=w541:cdb[], "dz/domega out"=w540:cdb[])  [unwired: 9 in, 5 out]
            n316 = local write "cursor x selector"(w521) -> ()
            n317 = call "nanocal -- publish -- freq scan V2.vi"("publisher action"=publisher_action."set", "dz/dω IN (V)"=w540, "z IN (V)"=w541, "ω IN (Hz)"=w542) -> ()  [unwired: 5 in, 3 out]
          }
          frame "action: save freq scan" {
            n318 = local read "Freq sweep name template"() -> (w597:T8)
            n319 = call "MFLI -- publish -- freq scan.vi"("publisher action"=publisher_action."get") -> ("Voltage out (V)"=w593:cdb[], "Freq out (Hz)"=w594:dbl[])  [unwired: 9 in]
            n320 = call "filename-manage.vi"("filename pattern"=w597, "filename-action"=filename-action."uniquenum", "folder IN"="Save folder", "file name IN"="freq sweep file name") -> ("filename OUT"=w596:string)  [unwired: 5 in, 2 out]
            n321 = call "KM_appendline -- freq sweep.vi"("freq"=w594, "Vout(V)"=w593, "Save frequency scan"="Save folder", "read/write control"=KM_file_--_read-write_control."append one line", "name or relative path"=w596) -> ()  [unwired: 15 in]
            n322 = local write "freq sweep file name"(w596) -> ()
          }
          frame "action: fit" {
          }
          frame "void", Default {
          }
        }
      }
    }
  }
  n323 = call "replace cursor - plot ref - V2.vi"("Plot ref in"=w5, "new X"=w4, "new  Y"=w4, "cursor index"=2, "cursor action"=cursor_action."write") -> ()  [unwired: 11 in, 4 out]
  n324 = local write "newton pause"(w1) -> ()
  n325 = control-ref of="Plot:  colors"() -> (w2:refnum<vi>)
  n326 = while "interface" {
    tunnel: w21 -> [w605]
    tunnel: w9 -> [w604]
    tunnel: w5 -> [w602]
    tunnel: w2 -> [w601]
    tunnel: w1 -> [_]
    stop <- w603 stop-if-true
    n327 = event shown="[16] \"pause! :\": Value Change" {
      selector: w605 -> [_ _ _ _ _ _ _ _ _ _ _ _ _ _ _ _ _ _ _ _ _ _ _ _]
      dyn-events: _ -> [_ _ _ _ _ _ _ _ _ _ _ _ _ _ _ _ _ _ _ _ _ _ _ _]
      timeout: _ -> [_ _ _ _ _ _ _ _ _ _ _ _ _ _ _ _ _ _ _ _ _ _ _ _]
      tunnel: w604 -> [w606 _ w618 w620 _ w649 w651 w654 w659 w660 w662 w664 w667 _ w673 w713 _ w741 w744 w747 w750 w753 w763 _]
      tunnel: [_ _ _ _ _ _ _ _ "load! :l" _ _ _ _ _ _ _ _ _ _ _ _ _ _ _] -> _
      tunnel: [_ _ _ _ _ _ _ _ _ _ _ _ _ _ _ _ _ _ _ _ _ _ _ w767] -> w603
      tunnel: [_ _ _ _ _ "go! :" _ _ _ _ _ _ "parse! :p" _ _ _ "pause! :" "uco! :u" "math -->   τ's !" "τ's --> math!" "math --> string!" "string --> math!" _ _] -> _
      tunnel: w602 -> [_ _ _ _ _ _ _ _ _ _ _ _ _ _ w669 _ _ _ _ _ _ _ _ _]
      tunnel: w601 -> [_ _ _ _ _ _ _ _ _ _ _ _ _ _ _ w736 _ _ _ _ _ _ _ _]
      event "Plot: sweep window": Cursor Move {
        n328 = event-data() -> ("CursIdx"=w607:i32)  [unwired: 1 in]
        n329 = case shown="0..2" w607 {
          tunnel: w606 -> [w609 _]
          frame 0..2 {
            w608 = "action: fit"  # action
            n330 = Generate User Event(user event=w609, event data cluster=w608) -> ()  [unwired: 2 in, 2 out]
          }
          frame 3..5, Default {
          }
        }
      }
      event "scale gauge: Plot: complex plane": Value Change {
        n331 = event-data() -> ()  [unwired: 1 in, 1 out]
        n332 = local read "scale gauge: Plot: complex plane"() -> (w616:dbl)
        n333 = control-ref of="Plot: sweep window"() -> (w615:refnum<vi>)
        n334 = Multiply(x=w616, y=0.3) -> (x*y=w617:dbl)
        n335 = Bundle By Name(cluster=T18 {"window y"=0.0021014740628288917, "center x"=44850.89441339177, "center y"=2.5658109925320947, "window x"=17480.201988350764} ("window IN"), "window x"=w616, "window y"=w616, "center x"=w617, "center y"=0.0) -> (w614:T18)
        n336 = call "replace cursor - plot ref - V2.vi"("Plot ref in"=w615, "window IN"=w614, "cursor action"=cursor_action."zoom to win") -> ()  [unwired: 13 in, 4 out]
      }
      event "ζ", "T1", "τS", "τN", "τC", "κ0": Value Change {
        n337 = event-data() -> ()  [unwired: 1 in, 1 out]
        n338 = Generate User Event(user event=w618, event data cluster="action: new sweep" ("event data")) -> ()  [unwired: 2 in, 2 out]
      }
      event Value Change {
        n339 = event-data() -> ()  [unwired: 1 in, 6 out]
        n340 = Generate User Event(user event=w620, event data cluster="action: update enums" ("event data")) -> ()  [unwired: 2 in, 2 out]
      }
      event "ω0 (rad/sec)": Value Change {
        n341 = event-data() -> ()  [unwired: 1 in, 1 out]
        n342 = call "nanocal -- publish -- freq scan V2.vi"("publisher action"=publisher_action."get") -> ("z out (V)"=w647:cdb[], "ω out (Hz)"=w642:dbl[])  [unwired: 8 in, 1 out]
        n343 = control-ref of="Plot: sweep window"() -> (w629:refnum<vi>)
        n344 = local read "T1"() -> (w631:dbl)
        n345 = local read "τN"() -> (w633:dbl)
        n346 = local read "ζ"() -> (w630:dbl)
        n347 = local read "τS"() -> (w632:dbl)
        n348 = local read "τC"() -> (w634:dbl)
        n349 = local read "κ0"() -> (w635:dbl)
        n350 = Divide(x="ω0 (rad/sec)", y=6.283185307179586) -> (x/y=w640:dbl)
        n351 = call "3-lorentzian-heat-response.vi"("zeta"=w630, "T1"=w631, "tauS"=w632, "tauN"=w633, "tauC"=w634, "kappa0"=w635, "omega (rad/sec)"="ω0 (rad/sec)", "action"=3-lorentzian-heat-response_action."calc R") -> ("Romega"=w638:cdb)  [unwired: 7 in, 4 out]
        n352 = Complex To Re/Im(x + iy=w638) -> (x=w636:dbl, y=w637:dbl)
        n353 = Threshold 1D Array(2:w640, 3:w642) -> (0:w641:dbl)  [unwired: 1 in]
        n354 = call "replace cursor - plot ref - V2.vi"("Plot ref in"=w629, "new X"=w636, "new  Y"=w637, "cursor index"=0, "cursor action"=cursor_action."write") -> ("Plot ref out"=w643:refnum<vi>)  [unwired: 11 in, 3 out]
        n355 = Index Array(array=w647, index=w641) -> (element=w644:cdb)
        n356 = Complex To Re/Im(x + iy=w644) -> (x=w645:dbl, y=w646:dbl)
        n357 = call "replace cursor - plot ref - V2.vi"("Plot ref in"=w643, "new X"=w645, "new  Y"=w646, "cursor index"=1, "cursor action"=cursor_action."write") -> ()  [unwired: 11 in, 4 out]
      }
      event "go! :": Value Change {
        n358 = event-data() -> ()  [unwired: 1 in, 6 out]
        n359 = Generate User Event(user event=w649, event data cluster="action: gradient step" ("event data")) -> ()  [unwired: 2 in, 2 out]
      }
      event "select B (T)", "select θ (deg)", "ignore T !", "select T (T)", "ignore B !", "ignore θ !": Value Change {
        n360 = event-data() -> ()  [unwired: 1 in, 6 out]
        n361 = Generate User Event(user event=w651, event data cluster="action: replot colors" ("event data")) -> ()  [unwired: 2 in, 2 out]
      }
      event "Plot: sweep window": Cursor Release {
        n362 = event-data() -> ("CursIdx"=w653:i32)  [unwired: 1 in, 8 out]
        n363 = case shown="0..2" w653 {
          tunnel: w654 -> [_ w655]
          frame 3, Default {
          }
          frame 0..2 {
            w656 = "action: fit"  # event data
            n364 = Generate User Event(user event=w655, event data cluster=w656) -> ()  [unwired: 2 in, 2 out]
          }
        }
      }
      event "load! :l": Value Change {
        n365 = event-data() -> ()  [unwired: 1 in, 6 out]
        n366 = Generate User Event "action User Event"(user event=w659, event data cluster="action: read from file" ("event data")) -> ()  [unwired: 2 in, 2 out]
      }
      event "Read from file": Value Change {
        n367 = event-data() -> ()  [unwired: 1 in, 6 out]
        n368 = Generate User Event "action User Event"(user event=w660, event data cluster="action: read from file" ("event data")) -> ()  [unwired: 2 in, 2 out]
      }
      event "off\nRe\nIm": Value Change {
        n369 = event-data() -> ()  [unwired: 1 in, 6 out]
        n370 = Generate User Event "action User Event"(user event=w662, event data cluster="action: read from file" ("event data")) -> ()  [unwired: 2 in, 2 out]
      }
      event "cspan": Value Change {
        n371 = event-data() -> ()  [unwired: 1 in, 6 out]
        n372 = Generate User Event "action User Event"(user event=w664, event data cluster="action: read from file" ("event data")) -> ()  [unwired: 2 in, 2 out]
      }
      event "parse! :p": Value Change {
        n373 = event-data() -> ()  [unwired: 1 in, 6 out]
        n374 = Generate User Event "action User Event"(user event=w667, event data cluster="action: parse string" ("event data")) -> ()  [unwired: 2 in, 2 out]
      }
      event Value Change {
        n375 = event-data() -> ()  [unwired: 1 in, 1 out]
      }
      event Key Down {
        n376 = event-data() -> ("Char"=w671:i16, "VKey"=w674:T19)  [unwired: 1 in]
        n377 = Build Array(w671) -> (w672:i16[])
        n378 = Byte Array To String(unsigned byte array=w672) -> (string=w670:string)
        n379 = case shown="\"ASCII\", Default" w674 {
          selector: w674 -> [_ _ _ _ _ w706]
          tunnel: w673 -> [w677 _ _ w702 _ _]
          tunnel: w670 -> [w676 _ _ _ _ _]
          tunnel: w669 -> [w675 _ _ _ _ w705]
          frame "ASCII", Default {
            n380 = case shown="\"+\", \",\", \"-\", \".\", \"<\", \"=\", \">\"" w676 {
              selector: w676 -> [_ _ _ _ _ _ w689 _ _ _ _]
              tunnel: w677 -> [_ _ w678 w680 w683 _ _ _ w696 w698 w700]
              tunnel: w675 -> [_ _ _ _ _ w687 _ _ _ _ _]
              frame "0", Default {
              }
              frame "a" {
              }
              frame "s" {
                n381 = Generate User Event(user event=w678, event data cluster="action: save freq scan" ("event data")) -> ()  [unwired: 2 in, 2 out]
              }
              frame "l" {
                n382 = Generate User Event(user event=w680, event data cluster="action: read from file" ("event data")) -> ()  [unwired: 2 in, 2 out]
              }
              frame " " {
                n383 = Generate User Event(user event=w683, event data cluster="action: gradient step" ("event data")) -> ()  [unwired: 2 in, 2 out]
              }
              frame "?" {
                # "?"
                n384 = call "replace cursor - plot ref - V2.vi"("Plot ref in"=w687, "cursor action"=cursor_action."zoom to win") -> ("Plot ref out"=w686:refnum<vi>)  [unwired: 14 in, 3 out]
                n385 = call "replace cursor - plot ref - V2.vi"("Plot ref in"=w686, "cursor action"=cursor_action."smart zoom out&aspect") -> ()  [unwired: 14 in, 4 out]
              }
              frame "+", ",", "-", ".", "<", "=", ">" {
                n386 = local read "step"() -> (w691:dbl)
                n387 = case shown="\"0\", Default" w689 {
                  tunnel: [0.7 1.0 1.5] -> w688
                  frame ",", "-", "<" {
                  }
                  frame "0", Default {
                  }
                  frame "+", ".", "=", ">" {
                  }
                }
                n388 = Multiply(x=w688, y=w691) -> (x*y=w690:dbl)
                n389 = local write "step"(w690) -> ()
              }
              frame "b" {
                n390 = local read "String"() -> (w695:string)
                n391 = local write "backup string :b"(w695) -> ()
              }
              frame "u" {
                n392 = Generate User Event(user event=w696, event data cluster="ignoreaction: uco" ("event data")) -> ()  [unwired: 2 in, 2 out]
              }
              frame "p" {
                n393 = Generate User Event "action User Event"(user event=w698, event data cluster="action: parse string" ("event data")) -> ()  [unwired: 2 in, 2 out]
              }
              frame "m" {
                n394 = Generate User Event "action User Event"(user event=w700, event data cluster="action: copy from math" ("event data")) -> ()  [unwired: 2 in, 2 out]
              }
            }
          }
          frame "Escape" {
          }
          frame "PageUp" {
          }
          frame "Enter" {
            n395 = Generate User Event "action User Event"(user event=w702, event data cluster="action: replot colors" ("event data")) -> ()  [unwired: 2 in, 2 out]
            n396 = Generate User Event "action User Event"(user event=w702, event data cluster="action: new sweep" ("event data")) -> ()  [unwired: 2 in, 2 out]
          }
          frame "PageDown" {
          }
          frame "Up".."Right" {
            n397 = case shown="\"Down\"" w706 {
              tunnel: [cursor_action."zoom in 20%" ("cursor action") cursor_action."zoom out 20%" ("cursor action") cursor_action."zoom out 20%" ("cursor action") cursor_action."zoom in 20%" ("cursor action")] -> w707
              frame "Up", Default {
              }
              frame "Down" {
              }
              frame "Left" {
              }
              frame "Right" {
              }
            }
            n398 = call "replace cursor - plot ref - V2.vi"("Plot ref in"=w705, "cursor action"=w707) -> ()  [unwired: 14 in, 4 out]
          }
        }
      }
      event "Plot:  colors": Cursor Move {
        n399 = event-data() -> ("CursIdx"=w715:i32)  [unwired: 1 in]
        n400 = local read "T1"() -> (w731:dbl)
        n401 = local read "τS"() -> (w732:dbl)
        n402 = local read "τN"() -> (w733:dbl)
        n403 = local read "τC"() -> (w734:dbl)
        n404 = local read "κ0"() -> (w735:dbl)
        n405 = local read "ζ"() -> (w730:dbl)
        n406 = call "replace cursor - plot ref - V2.vi"("Plot ref in"=w736, "cursor index"=w715, "cursor action"=cursor_action."read") -> ("read Y"=w714:dbl)  [unwired: 13 in, 3 out]
        n407 = Build Array(w730, w731, w732, w733, w734, w735) -> (w717:dbl[])
        n408 = Replace Array Subset(array=w717, new element=w714, index=w715) -> (w716:dbl[])
        n409 = Generate User Event(user event=w713, event data cluster="action: replot circles" ("event data")) -> ()  [unwired: 2 in, 2 out]
        n410 = Index Array(array=w716, index #1=0 ("index"), index #2=1 ("index"), index #3=2 ("index"), index #4=3 ("index"), index #5=4 ("index"), index #6=5 ("index")) -> (element #1=w723:dbl, element #2=w722:dbl, element #3=w721:dbl, element #4=w720:dbl, element #5=w719:dbl, element #6=w718:dbl)
        n411 = local write "τN"(w720) -> ()
        n412 = local write "τC"(w719) -> ()
        n413 = local write "τS"(w721) -> ()
        n414 = local write "κ0"(w718) -> ()
        n415 = local write "T1"(w722) -> ()
        n416 = local write "ζ"(w723) -> ()
      }
      event "pause! :": Value Change {
        n417 = event-data() -> ()  [unwired: 1 in, 6 out]
        n418 = local write "newton pause"(TRUE ("newton pause")) -> ()
      }
      event "uco! :u": Value Change {
        n419 = event-data() -> ()  [unwired: 1 in, 1 out]
        n420 = Generate User Event(user event=w741, event data cluster="ignoreaction: uco" ("event data")) -> ()  [unwired: 2 in, 2 out]
      }
      event "math -->   τ's !": Value Change {
        n421 = event-data() -> ()  [unwired: 1 in, 1 out]
        n422 = Generate User Event(user event=w744, event data cluster="action: copy from math" ("event data")) -> ()  [unwired: 2 in, 2 out]
      }
      event "τ's --> math!": Value Change {
        n423 = event-data() -> ()  [unwired: 1 in, 1 out]
        n424 = Generate User Event(user event=w747, event data cluster="action: copy to math" ("event data")) -> ()  [unwired: 2 in, 2 out]
      }
      event "math --> string!": Value Change {
        n425 = event-data() -> ()  [unwired: 1 in, 1 out]
        n426 = Generate User Event(user event=w750, event data cluster="action: write mathematica string" ("event data")) -> ()  [unwired: 2 in, 2 out]
      }
      event "string --> math!": Value Change {
        n427 = event-data() -> ()  [unwired: 1 in, 1 out]
        n428 = Generate User Event(user event=w753, event data cluster="action: read mathematica string" ("event data")) -> ()  [unwired: 2 in, 2 out]
      }
      event "filenames": Value Change {
        n429 = event-data() -> ()  [unwired: 1 in, 6 out]
        n430 = local read "filesnames lookup"() -> (w761:map{i32, i32})
        n431 = local read "filenames"() -> (w759:map{i32, string})
        n432 = local read "filenames"() -> (w760:u16)
        n433 = local read "folder"() -> (w762:path)
        n434 = Look In Map(map=w761, key=w760) -> (value=w758:i32)  [unwired: 1 in, 1 out]
        n435 = Look In Map(map=w759, key=w758) -> (value=w757:string)  [unwired: 1 in, 1 out]
        n436 = Build Path(base path=w762, name or relative path=w757) -> (appended path=w755:path)
        n437 = for {
          N: 1 -> [_]
          tunnel: w763 -> [w765]
          tunnel: w755 -> [w764]
          n438 = local write "Read from file"(w764) -> ()
          n439 = Generate User Event(user event=w765, event data cluster="action: read from file" ("event data")) -> ()  [unwired: 2 in, 2 out]
        }
      }
      event User Event {
        n440 = event-data() -> ("interface"=w768:string)  [unwired: 1 in, 4 out]
        n441 = case shown="\"False\", Default" w768 {
          tunnel: [_ TRUE] -> w767
          frame "False", Default {
          }
          frame "interface: exit" {
          }
        }
      }
    }
  }
  "cursor x selector" <- w3
